vi "Main.vi"() -> ()   [LabVIEW 2013]
uses:
  Control 1.ctl
  Moteurs PI/PI Controls/Type de Mouvement PI.ctl
  Moteurs PI/PI Controls/AxeADeplacer.ctl
  PilMOT/Controls/Axes.ctl
  Commandes/Type de Mouvement PilMOT.ctl
  Moteurs PI/PI Globals/Zero.vi
panel:
  out "INIT":bool caption="En cours..."
  in  "CLR ERR mot PI 2":bool
  out "error out \nPI Enceinte 2":errorcluster
  in  "Fichier Fins de Courses":path=path "C:/Users/appli/Documents/Manip Gaz/Moteurs manip Gaz - Multithread/PilMOT/RefsMoteurs/FDC.dat"
  in  "CLR ERR mot PI":bool
  out "error out \nPI Enceinte":errorcluster
  in  "CLR ERR LàR":bool
  out "error out\nLabview functions":errorcluster
  in  "Fichier zéro ligne à retard":path=path "C:/Users/appli/Documents/Manip Gaz/Moteurs manip Gaz - Multithread/Moteurs PI/PI Globals/zero.dat"
  out "error out \nligne à retard":errorcluster
  in  "stop":bool
  out "error out\nesbim":cluster{"status":bool, "code":i32, "source":T1}
  in  "Commande onglets":T2(tab)
  in  "Axes\nà ref. 2":string[](array[string])=["1", "2", "3", "4"]
  in  "Modèles des platines":string[](array[string])=["M-111.1VG ", "M-111.1VG ", "M-111.1VG ", "M-111.1VG "]
  in  "Referencing":T3={"Check FRF?"=TRUE, "Referencing mode"=[enum."FPL", enum."FPL", enum."FPL", enum."FPL", enum."FRF (-> FNL)", enum."FRF (-> FNL)"]}
  out "Referencing...":bool caption="En cours..."
  in  "Limit switch selection":u16[](array[ring]) items=["Positive (MPL)", "Negative (MNL)"]
  out "Host address":string
  out "Referencing\nsuccessful?":bool[](array[boolean])
  in  "Ref tous\nles axes? 2":bool=TRUE
  out "Amplitude \n (+/-) (mm) 2":dbl[](array[numeric]) format="%.6f"
  out "Position 2":dbl[](array[numeric]) format="%.6f"
  out "Referencing...":bool
  out "Etat moteurs PI Buse/Capillaire 2":string
  out "Axes \nConn. 2":string[](array[string])
  in  "Configurer moteurs Enceinte (PI) 2":bool
  out "Identification C884":string
  out "En cours... 2":bool
  in  "Configurer Mercury (PI)":bool
  out "Etat moteurs PI Capillaire/Objectif":string
  in  "Configurer moteurs Enceinte (PI)":bool
  out "Identification carte de contrôle":string
  out "Axes \nConn.":string[](array[string])
  out "Amplitude \ndu mouvement\npermise (+/-) (mm)":dbl[](array[numeric]) format="%.6f"
  in  "Déplacement \nmi-course?":bool
  in  "Axes\nà ref.":string[](array[string])=["1", "2", "3", "4"]
  in  "Ref tous\nles axes?":bool
  out "Position":dbl[](array[numeric]) format="%.6f"
  out "+/- movement\nrange":dbl[](array[numeric]) format="%.6f"
  out "Position ligne à retard":dbl[](array[numeric]) format="%.6f"
  out "Conn. \nAxes":string[](array[string])
  out "Identification":string
  out "Etat ligne à retard":string
  in  "Stage selection":T4
  out "Axes \nConnectés\n(PI)  2":string[](array[string])
  in  "Positions de référence 2":dbl[][](array[numeric])=[[0.0, 0.0, 0.0, 0.0], [0.0, 0.0, 0.0, 0.0], [0.0, 0.0, 0.0, 0.0], [0.0, 0.0, 0.0, 0.0]] format="%_7g"
  out "Axes \nConnectés\n(PI)":string[](array[string])
  in  "SafeMax 2":dbl[](array[numeric]) format="%.6f"
  in  "SafeMin 2":dbl[](array[numeric]) format="%.6f"
  in  "SafeMax 1":dbl[](array[numeric]) format="%.6f"
  in  "SafeMin 1":dbl[](array[numeric]) format="%.6f"
  out "Axe en MVT 2":bool[](array[boolean])
  out "Position Moteurs (PI) 2":dbl[](array[numeric]) format="%.6f"
  in  "Déplacement (mm) 2":dbl[](array[numeric]) format="%.6f"
  in  "Axes à déplacer \n(PI) 2":bool[](array[boolean])
  out "Initialisation OK? 2":bool
  out "Axe en MVT":bool[](array[boolean])
  in  "Stop Mvt":bool
  in  "Axe (PI refs)":T5
  in  "Axe à déplacer (PI)":T5
  in  "MVT+":bool
  in  "MVT-":bool
  in  "Référence":T6(ring)
  in  "Positions de référence":dbl[][](array[numeric])=[[0.0, 0.0, 0.0, 0.0], [0.0, 0.0, 0.0, 0.0], [0.0, 0.0, 0.0, 0.0], [0.0, 0.0, 0.0, 0.0]] format="%_7g"
  in  "Load":bool
  in  "Save":bool
  in  "Go to Ref (PI)":bool
  in  "Set Ref (PI)":bool
  in  "Axes à déplacer \n(PI)":bool[](array[boolean])
  in  "Type de déplacement":T7
  out "Position Moteurs (PI)":dbl[](array[numeric]) format="%.6f"
  in  "Déplacement (mm)":dbl[](array[numeric]) format="%.6f"
  in  "Déplacer":bool
  in  "Déplacement":dbl[](array[numeric])=[0.001]
  out "Initialisation OK?":bool
  in  "Nom Fichier Refs PI":string="REFS"
  in  "Stop here":bool
  out "Current zero position":dbl
  in  "zero":dbl
  in  "zero à :":bool
  in  "zero ici":bool
  in  "JOG + delay":bool
  in  "Go delay":bool
  in  "JOG -delay":bool
  in  "Delay to reach":dbl
  in  "Step Size (ps)":dbl
  out "Ligne à retard prête?":bool
  in  "JOG + position":bool
  in  "Go pos":bool
  in  "JOG - position":bool
  in  "Query Pos.":bool
  in  "Position à atteindre":dbl
  in  "Step Size (mm)":dbl
  out "Position de la ligne à retard":dbl(slide) min=-51.0 max=51.0 scale=0.0..100.0
  in  "Query Velocity":bool
  in  "Set Vel.":dbl
  in  "Set Velocity":bool
  out "Current velocity":dbl
  out "Error Description (delay line)":string
  out "Initialisation OK?":bool
  in  "Axe à déplacer PilMot":T8=1 items=["Axe 1"=1, "Axe 2"=2, "Axe 3"=3, "Axe 4"=4, "Axe 5"=5, "Axe 6"=6]
  in  "Positions de référence PilMot":dbl[][](array[numeric])=[[0.0, 0.0, 0.0, 0.0], [0.0, 0.0, 0.0, 0.0], [0.0, 0.0, 0.0, 0.0], [0.0, 0.0, 0.0, 0.0]] format="%_7g"
  in  "Nom Fichier Refs PilMOT":string="StepperRef"
  out "Envoi cmde PilMot?":bool
  in  "STOP MOTEURS!!":bool
  in  "Coeff µm/pas":dbl[](array[numeric])=[3.1, 3.1, 3.1, 3.1, 3.1, 3.1]
  out "Positons Moteurs":dbl[](array[numeric])
  in  "Mouvement Rel/Abs":u16(ring) items=["Mouvement Absolu", "Mouvement Relatif"]
  in  "Origine":bool
  in  "Vitesses":i32[](array[numeric])=[0, 0, 0, 0, 0, 0]
  in  "Axes à déplacer \n(PilMot)":bool[](array[boolean])
  in  "Aller à CàA":bool
  in  "Axe à déplacer":u16(ring)=1 items=["Axe 1"=1, "Axe 2"=2, "Axe 3"=3, "Axe 4"=4, "Axe 5"=5, "Axe 6"=6]
  in  "Déplacement -":bool
  in  "Déplacement +":bool
  out "Adresse du PilMOT":string="ni.var.psp://localhost/OPC/OPC1/esbimETH_1"
  in  "Cotes à atteindre":dbl[](array[numeric])=[0.0, 0.0, 0.0, 0.0, 0.0, 0.0] format="%_6f"
  in  "Connected?":bool
  in  "Référence PilMot":T6(ring)
  in  "Set Ref (PilMot)":bool
  in  "Go to Ref (PilMot)":bool
  in  "Save Ref PilMot":bool
  in  "Load Ref PilMot":bool
  # "NE JAMAIS REFERENCER EN POSITION OBJECTIF"
  # "Objective Focus"
  # "Objective height"
  # "Target Height"
  # "<unassigned>"
  # "Target Transverse"
  # "Target  Focus"
  # "Mitu Obj Focus"
  # "Mitu Obj Transverse"
  # "FNL"
  # "FPL"
  # "FNL"
  # "FPL"
  # "Objective Focus"
  # "Objective height"
  # "Target Height"
  # "<unassigned>"
  # "Target Transverse"
  # "Target  Focus"
  # "Mitu Obj Focus"
  # "Mitu Obj Transverse"
  # "Objective Focus"
  # "Objective height"
  # "Target Height"
  # "<unassigned>"
  # "Target Transverse"
  # "Target  Focus"
  # "<unassigned>"
  # "<unassigned>"
  # "mm"
  # "mm"
  # "Spectro Electrons"
  # "NO MOTOR"
  # "Objectif/Jet"
  # "Pinhole Spectro"
  # "Parabole reprise"
  # "HeNe Salle Orange"
  # "Moteur 1"
  # "Spectro Electrons"
  # "Objectif/Jet"
  # "Pinhole Spectro"
  # "Parabole reprise"
  # "Moteur 6"
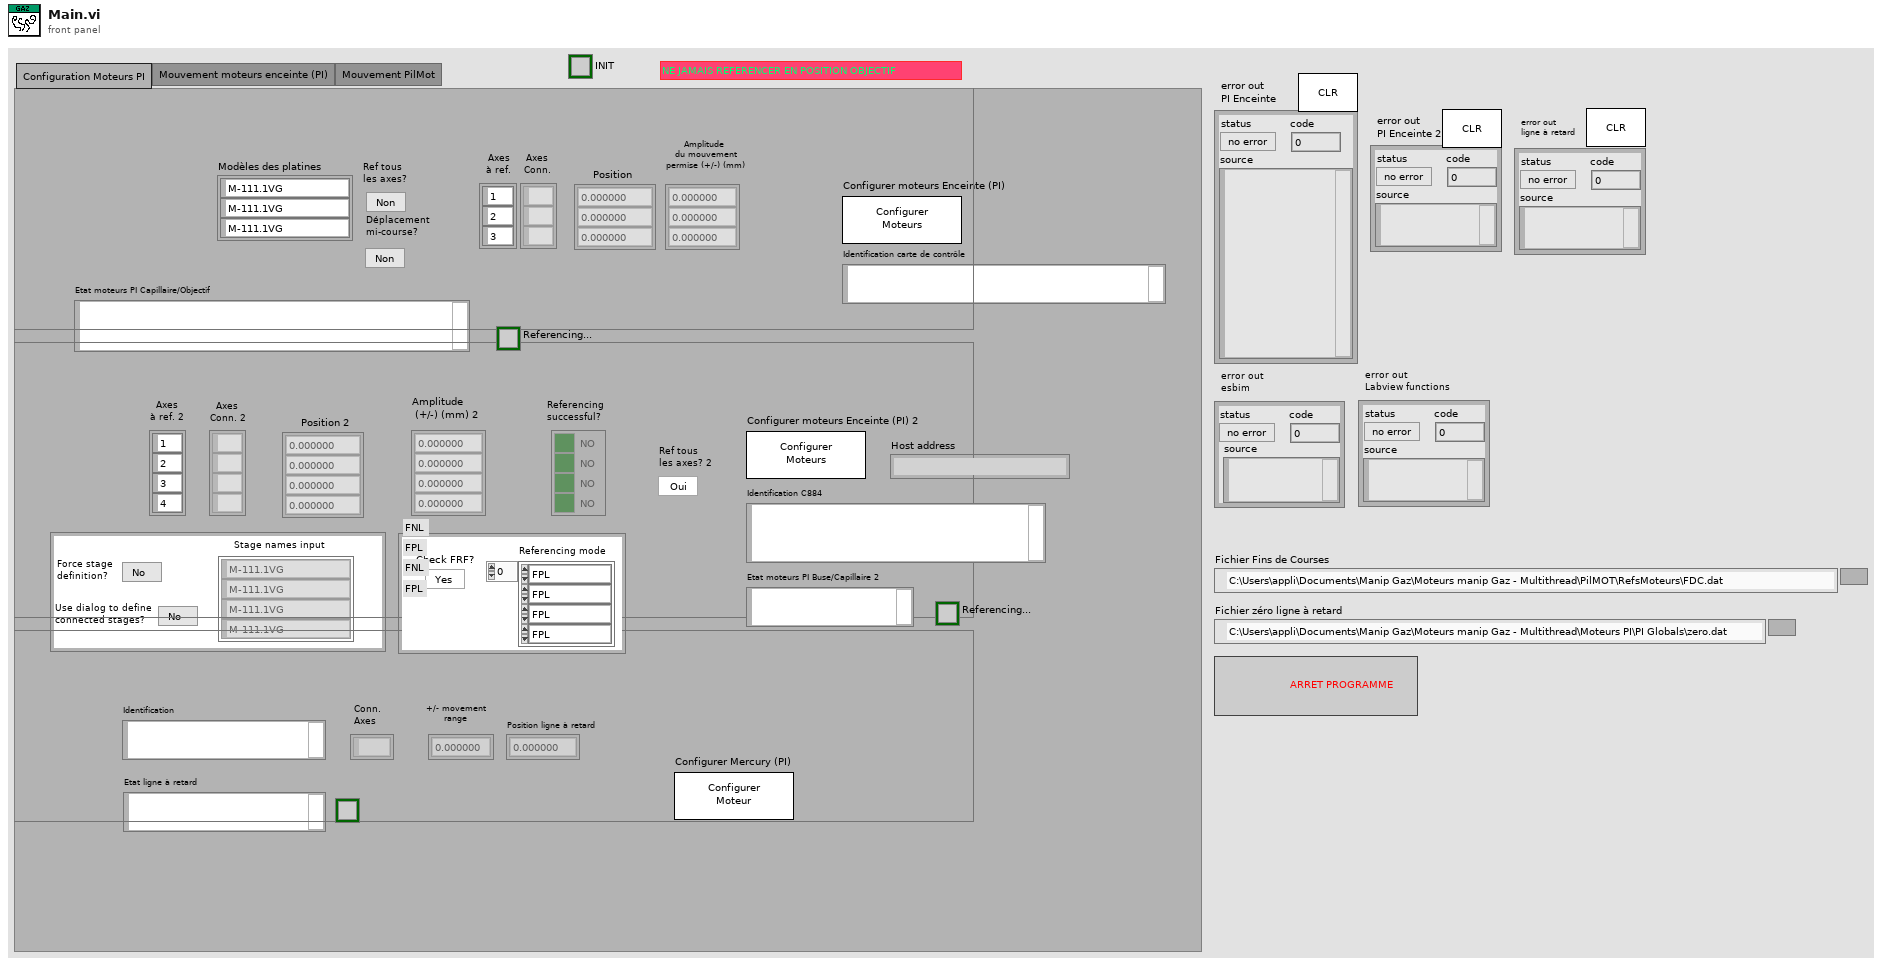
[diagram p1: front panel]
types:
  T1 = typedef "Control 1.ctl" = string
  T2 = enum32{"Configuration Moteurs PI", "Mouvement moteurs enceinte (PI)", "Mouvement Ligne à retard (PI)", "Mouvement PilMot"}
  T3 = cluster{"Check FRF?":bool, "Referencing mode":enum16{"FRF (-> FNL)", "FRF", "FNL", "FPL", "RON OFF"}[]}
  T4 = cluster{"Force?":bool, "Dialog?":bool, "Stages":string[]}
  T5 = typedef "AxeADeplacer.ctl" = enum16{"Objective Focus", "Objective Height", "Target Height", "<unassigned 1, 4>", "Target Transverse", "Target Focus", "Mitu Obj Focus", "Mitu Obj Transverse"}
  T6 = enum16{"Référence 1", "Référence 2", "Référence 3", "Référence 4"}
  T7 = typedef "Type de Mouvement PI.ctl" = enum16{"Mouvement absolu", "Mouvement relatif (-)", "Mouvement relatif (+)", "Définir pos. référence", "Aller à la pos. ref."}
  T8 = typedef "Axes.ctl" = u16
  T9 = enum16{"open", "replace", "create", "open or create", "replace or create", "replace or create with confirmation"}
  T10 = typedef "Type de Mouvement PilMOT.ctl" = u16
  T11 = typedef "AdressesVariablesPartagees.ctl" = cluster{"OrdreBloc":string, "Ordre UC":string, "CoteAAtteindre":string, "Vitesse":string, "Position codeur en pas":string, "Position Théorique":string, "Message":string, "Ecrire":string, "Zone à écrire":string, "Numéro paramètre":string, "Ordre":string, "Valeur":string, "Valeur Lecture":string, "Numéro paramètre Lecture":string, "Acquittement Lecture Ecriture":string, "Zone à Ecrire Pour Axe ":u16, "Acquittement Ordre UC":string}
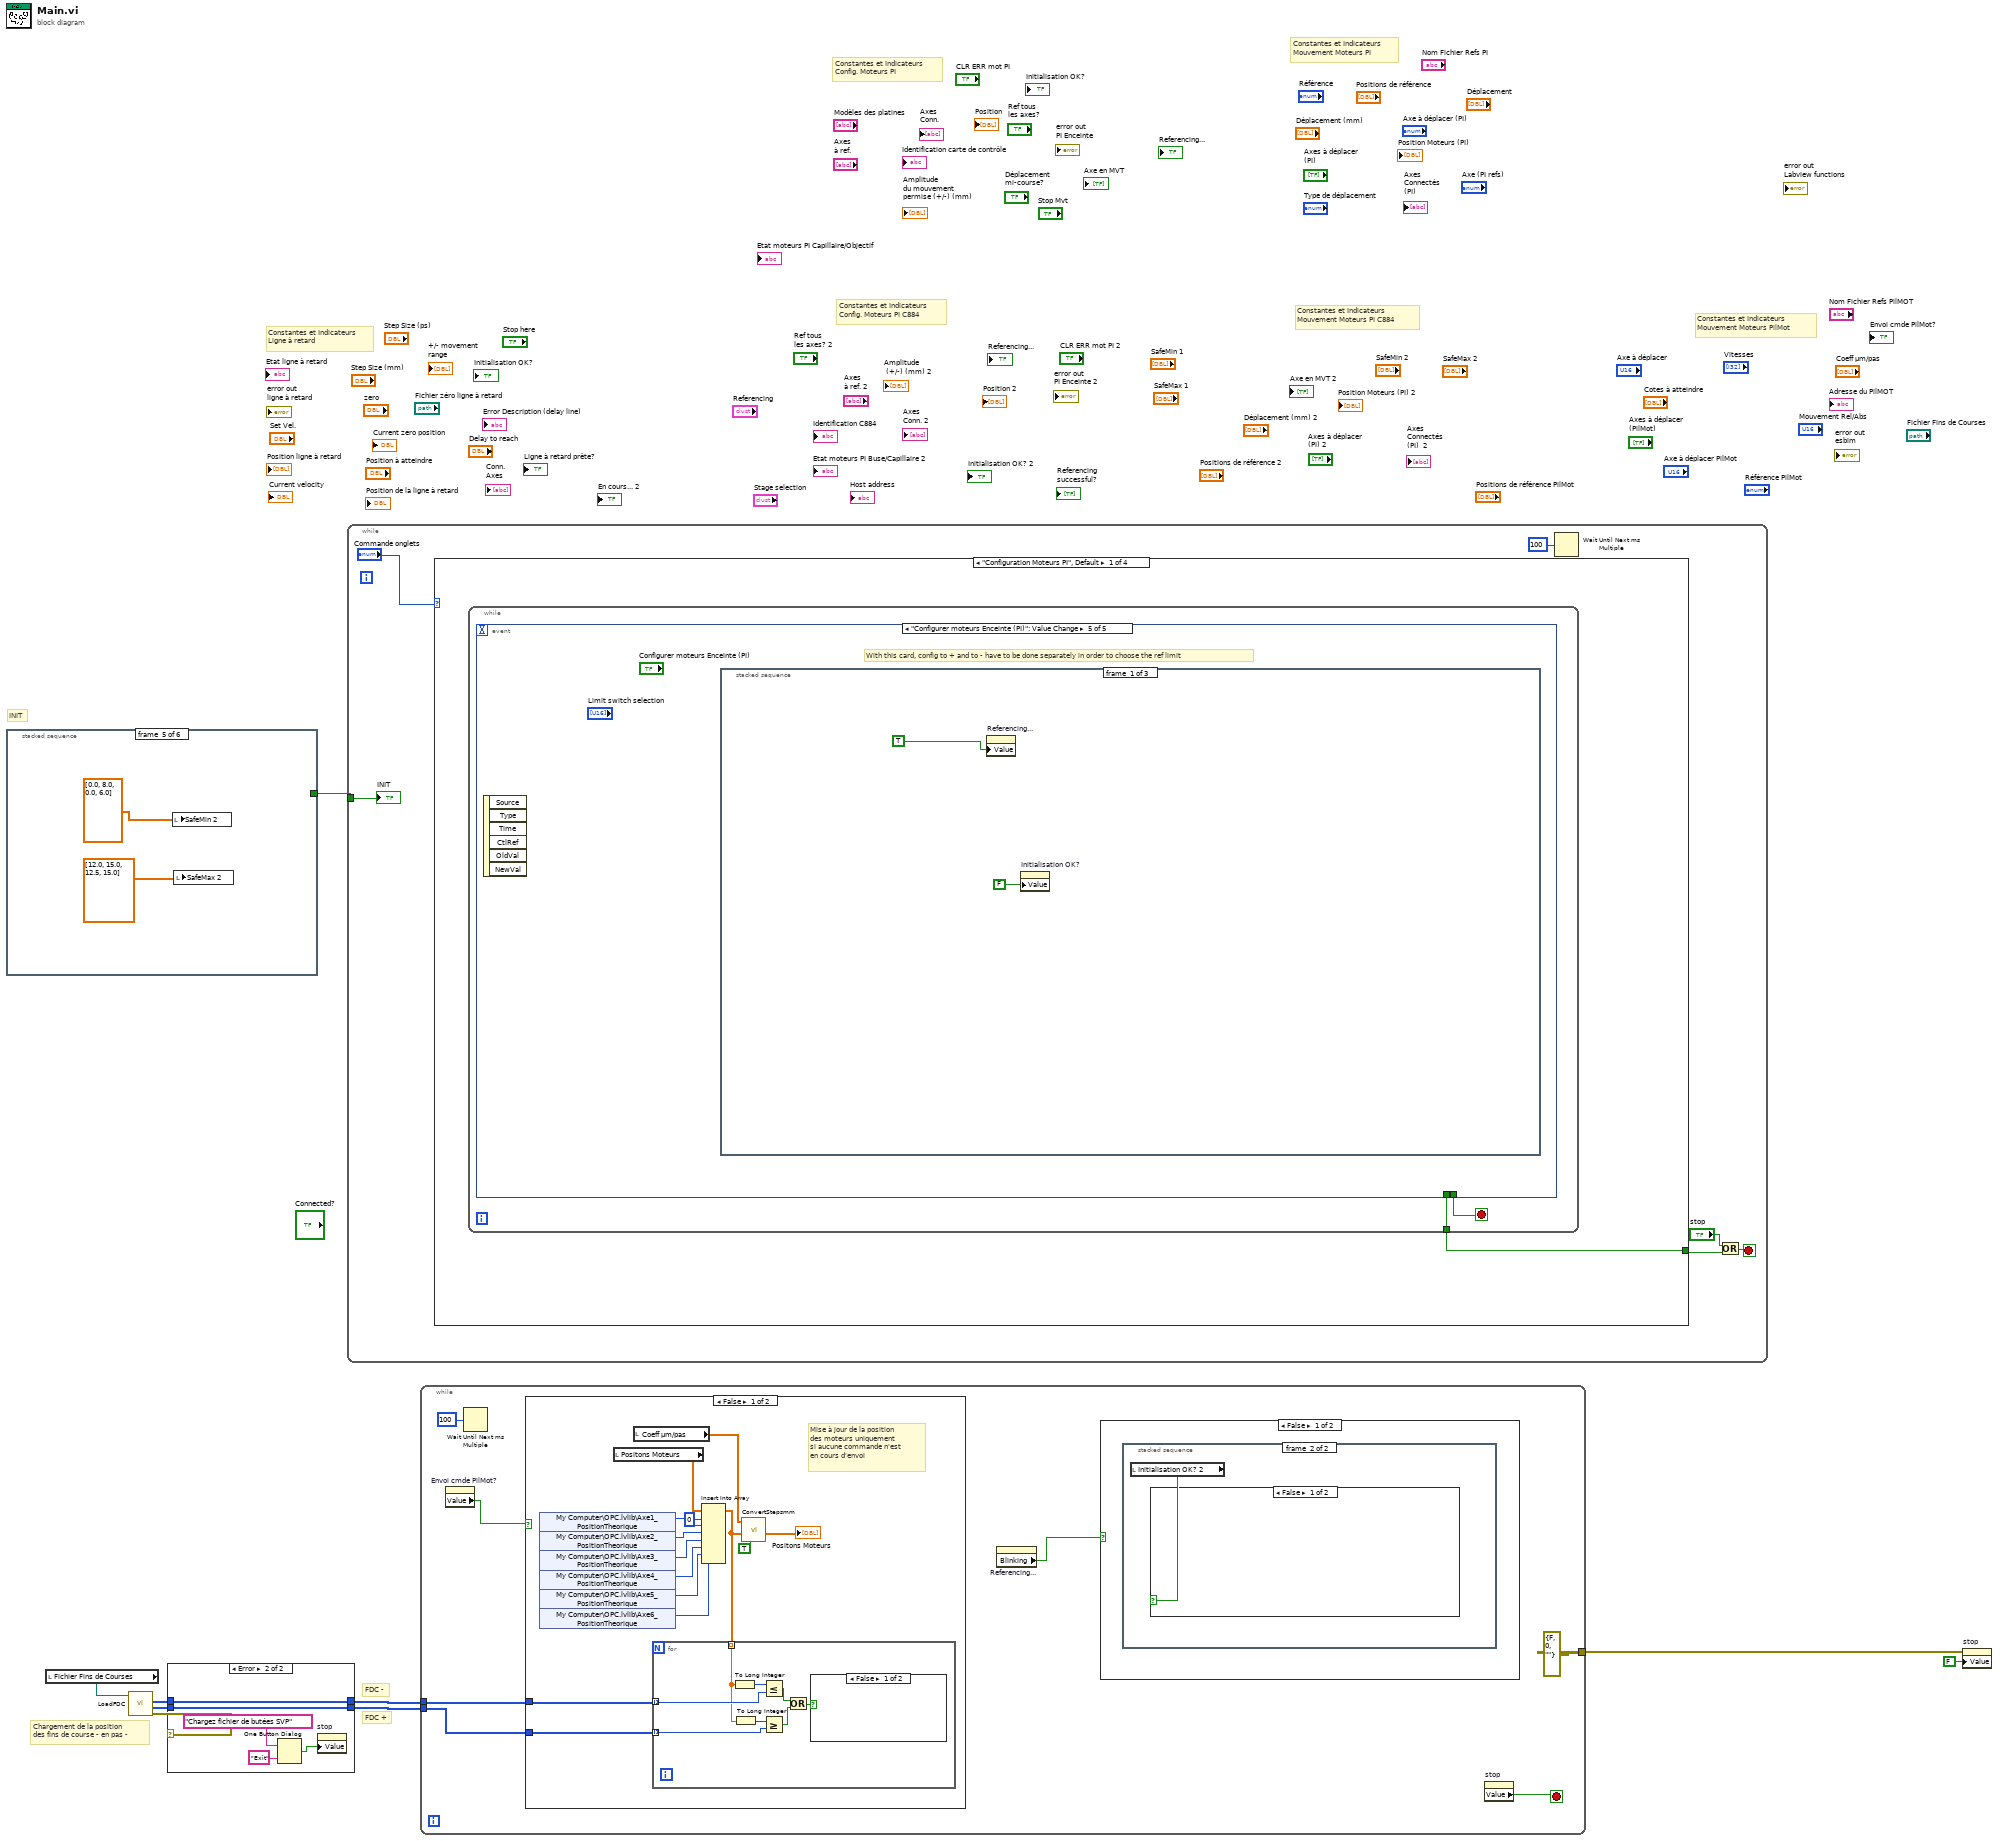
[diagram p0: block diagram]
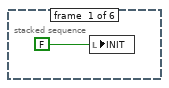
[diagram p2: hidden frame]
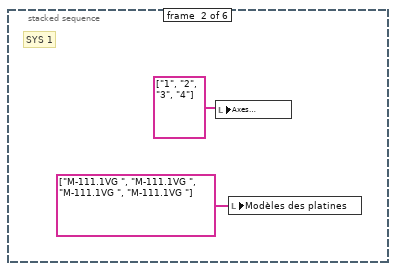
[diagram p3: hidden frame]
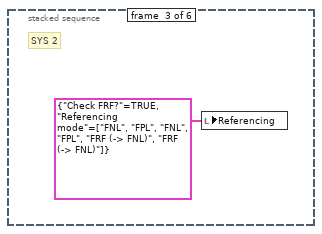
[diagram p4: hidden frame]
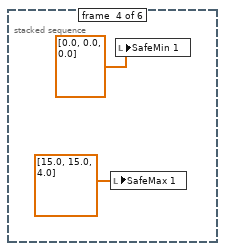
[diagram p5: hidden frame]
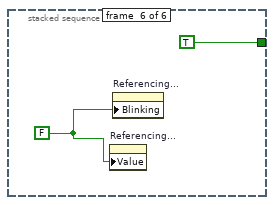
[diagram p6: hidden frame]
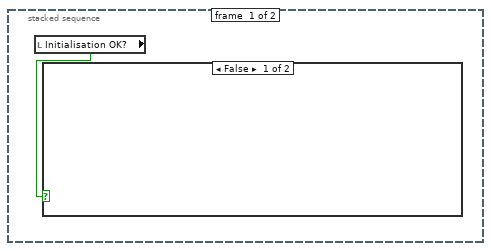
[diagram p8: hidden frame]
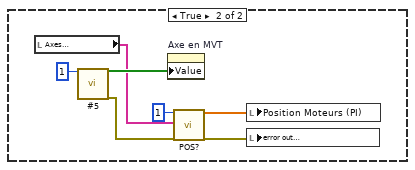
[diagram p9: hidden frame]
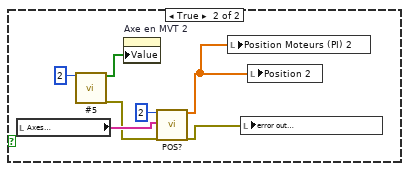
[diagram p10: hidden frame]
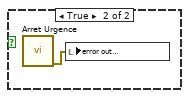
[diagram p12: hidden frame]
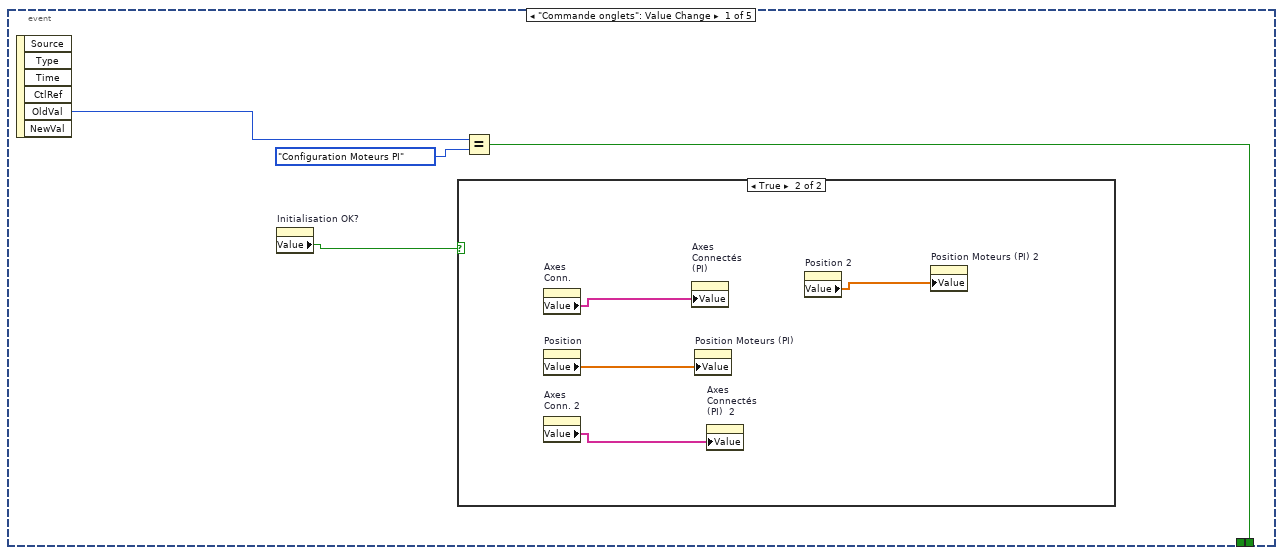
[diagram p14: hidden frame]
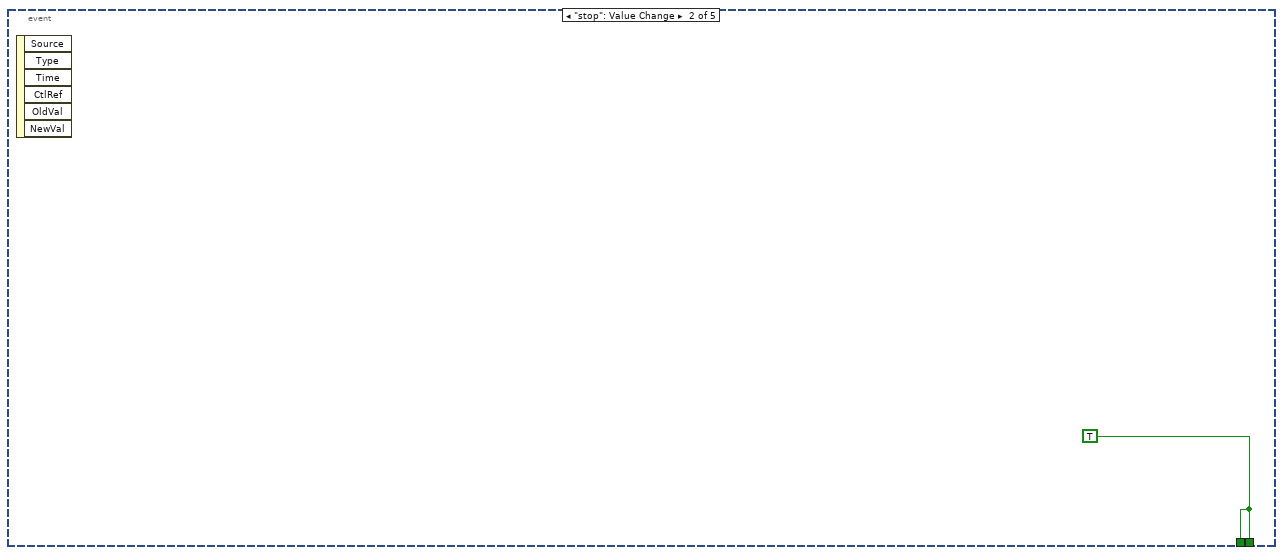
[diagram p16: hidden frame]
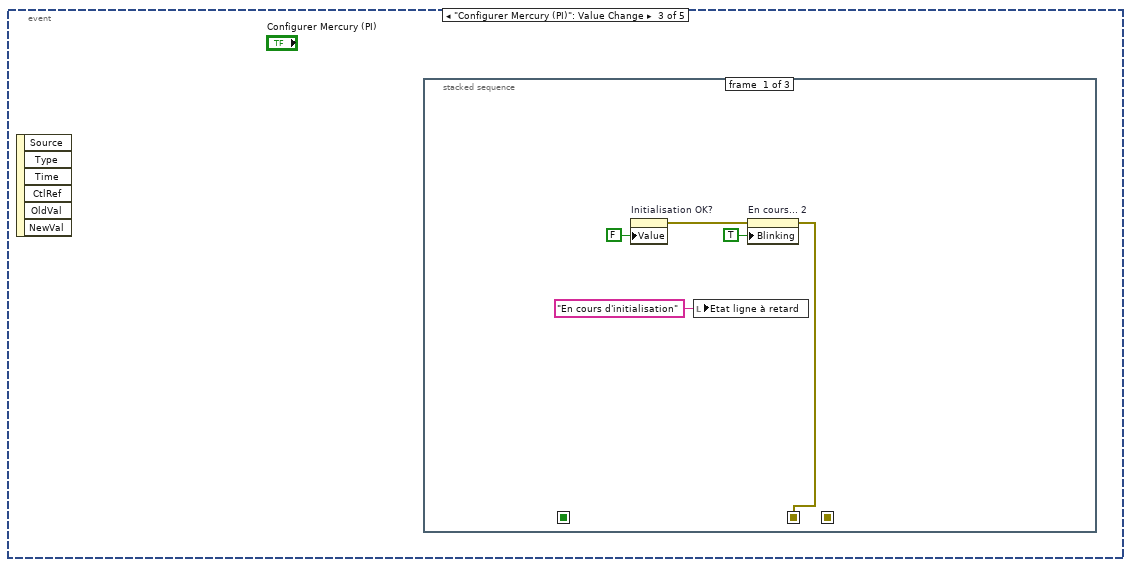
[diagram p17: hidden frame]
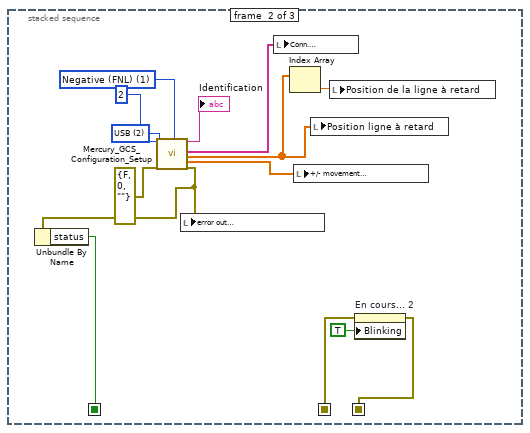
[diagram p18: hidden frame]
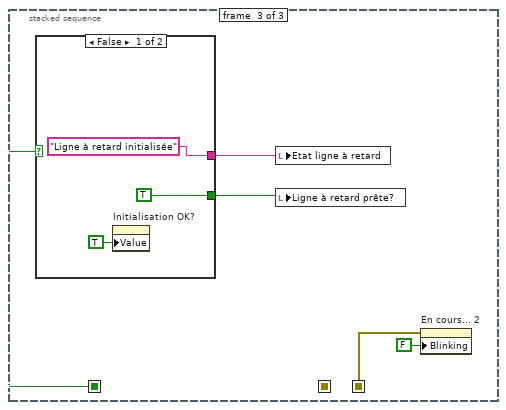
[diagram p19: hidden frame]
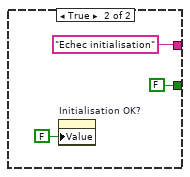
[diagram p20: hidden frame]
diagram:
  # "INIT"
  # "Constantes et Indicateurs\nMouvement Moteurs PI C884"
  # "Constantes et Indicateurs \nConfig. Moteurs PI C884"
  # "Chargement de la position \ndes fins de course - en pas -"
  # "FDC +"
  # "FDC -"
  # "Constantes et Indicateurs\nLigne à retard"
  # "Constantes et Indicateurs\nMouvement Moteurs PilMot"
  # "Constantes et Indicateurs\nMouvement Moteurs PI"
  # "Constantes et Indicateurs \nConfig. Moteurs PI"
  n1 = stacked-sequence {
    tunnel: [_ _ _ _ _ TRUE] -> w1
    frame #0 {
      n2 = local write "INIT"(FALSE) -> ()
    }
    frame #1 {
      # "SYS 1"
      n3 = local write "Axes\nà ref."(string[] ["1", "2", "3", "4"] ("Axes\nà ref.")) -> ()
      n4 = local write "Modèles des platines"(string[] ["M-111.1VG ", "M-111.1VG ", "M-111.1VG ", "M-111.1VG "] ("Modèles des platines")) -> ()
    }
    frame #2 {
      # "SYS 2"
      n5 = local write "Referencing"(T3 {"Check FRF?"=TRUE, "Referencing mode"=[enum."FNL", enum."FPL", enum."FNL", enum."FPL", enum."FRF (-> FNL)", enum."FRF (-> FNL)"]} ("Referencing")) -> ()
    }
    frame #3 {
      n6 = local write "SafeMax 1"(dbl[] [15.0, 15.0, 4.0] ("SafeMin 1")) -> ()
      n7 = local write "SafeMin 1"(dbl[] [0.0, 0.0, 0.0] ("SafeMin 1")) -> ()
    }
    frame #4 {
      n8 = local write "SafeMin 2"(dbl[] [0.0, 8.0, 0.0, 6.0] ("SafeMin 1")) -> ()
      n9 = local write "SafeMax 2"(dbl[] [12.0, 15.0, 12.5, 15.0] ("SafeMin 1")) -> ()
    }
    frame #5 {
      w18 = FALSE ("Blinking")
      n10 = property on="Referencing..." class="Bool (strict)"("Value"=w18) -> ()  [unwired: 2 in, 2 out]
      n11 = property on="Referencing..." class="Bool (strict)"("Blinking"=w18) -> ()  [unwired: 2 in, 2 out]
    }
  }
  n12 = local read "Fichier Fins de Courses"() -> (w7:path)
  n13 = call "LoadFDC.vi"("file path (use dialog)"=w7) -> ("error out"=w6:errorcluster, "FDC+"=w4:i32[], "FDC-"=w5:i32[])  [unwired: 8 in]
  n14 = case shown="Error" w6 {
    tunnel: w5 -> [w21 w26]
    tunnel: [w21 w26] -> w3
    tunnel: w4 -> [w20 w25]
    tunnel: [w20 w25] -> w2
    frame No Error {
    }
    frame Error {
      n15 = One Button Dialog(message="Chargez fichier de butées SVP", button name ("OK")="Exit") -> (true=w22:bool)
      n16 = property on="stop" class="Bool (strict)"("Value"=w22) -> ()  [unwired: 2 in, 2 out]
    }
  }
  n17 = while {
    tunnel: w1 -> [w27]
    stop <- w31 stop-if-true
    n18 = case shown="\"Configuration Moteurs PI\", Default" "Commande onglets" {
      tunnel: [w33 w123 w410 w577] -> w29
      frame "Configuration Moteurs PI", Default {
        n19 = while {
          tunnel: [w34] -> w33
          stop <- w35 stop-if-true
          n20 = event shown="[4] \"Configurer moteurs Enceinte (PI)\": Value Change" {
            selector: _ -> [_ _ _ _ _]
            dyn-events: _ -> [_ _ _ _ _]
            timeout: _ -> [_ _ _ _ _]
            tunnel: [w37 w44 _ _ _] -> w35
            tunnel: [_ w44 _ _ _] -> w34
            event "Commande onglets": Value Change {
              n21 = event-data() -> ("OldVal"=w39:T2)  [unwired: 1 in, 5 out]
              n22 = property on="Initialisation OK?" class="Bool (strict)"() -> ("Value"=w36:bool)  [unwired: 2 in, 2 out]
              n23 = case shown="True" w36 {
                frame False {
                }
                frame True {
                  n24 = property on="Axes \nConn." class="Arr (strict)"() -> ("Value"=w43:string[])  [unwired: 2 in, 2 out]
                  n25 = property on="Position" class="Arr (strict)"() -> ("Value"=w42:dbl[])  [unwired: 2 in, 2 out]
                  n26 = property on="Axes \nConn. 2" class="Arr (strict)"() -> ("Value"=w41:string[])  [unwired: 2 in, 2 out]
                  n27 = property on="Axes \nConnectés\n(PI)" class="Arr (strict)"("Value"=w43) -> ()  [unwired: 2 in, 2 out]
                  n28 = property on="Position Moteurs (PI)" class="Arr (strict)"("Value"=w42) -> ()  [unwired: 2 in, 2 out]
                  n29 = property on="Axes \nConnectés\n(PI)  2" class="Arr (strict)"("Value"=w41) -> ()  [unwired: 2 in, 2 out]
                  n30 = property on="Position 2" class="Arr (strict)"() -> ("Value"=w40:dbl[])  [unwired: 2 in, 2 out]
                  n31 = property on="Position Moteurs (PI) 2" class="Arr (strict)"("Value"=w40) -> ()  [unwired: 2 in, 2 out]
                }
              }
              n32 = Equal?(x=w39, y=T2."Configuration Moteurs PI" ("Commande onglets")) -> (x = y?=w37:bool)
            }
            event "stop": Value Change {
              w44 = TRUE
              n33 = event-data() -> ()  [unwired: 1 in, 6 out]
            }
            event "Configurer Mercury (PI)": Value Change {
              n34 = event-data() -> ()  [unwired: 1 in, 6 out]
              n35 = stacked-sequence {
                seq-local: [_ w57 _] -> [_ _ w68]
                seq-local: [w45 _ _] -> [_ w51 _]
                seq-local: [_ w50 _] -> [_ _ w64]
                frame #0 {
                  n36 = property on="Initialisation OK?" class="Bool (strict)"("Value"=FALSE ("Initialisation 2")) -> (error out=w46:errorcluster)  [unwired: 2 in, 1 out]
                  n37 = local write "Etat ligne à retard"("En cours d'initialisation" ("Etat ligne à retard")) -> ()
                  n38 = property on="En cours... 2" class="Bool (strict)"(error in=w46, "Blinking"=TRUE) -> (error out=w45:errorcluster)  [unwired: 1 in, 1 out]
                }
                frame #1 {
                  w60 = u16 1 items=["Positive (FPL)", "Negative (FNL)"] ("Limit switch selection")
                  w61 = u16 2 items=["RS232", "RS232 DaisyChain", "USB", "USB_DaisyChain"] ("Interface")
                  n39 = call "Mercury_GCS_Configuration_Setup.vi"("System no."=2, "Interface"=w61, "error in"=errorcluster {"status"=FALSE, "code"=0, "source"=""}, "Reference Move"=w60) -> ("Identification"=→"Identification":string, "Conn. \nAxes"=w56:string[], "Position"=w53:dbl[], "+/- movement\nrange"=w55:dbl[], "error out"=w58:errorcluster)  [unwired: 9 in, 2 out]
                  n40 = Unbundle By Name(w58) -> ("status"=w57:bool)
                  n41 = local write "error out \nligne à retard"(w58) -> ()
                  n42 = local write "Conn. \nAxes"(w56) -> ()
                  n43 = Index Array(array=w53) -> (element=w54:dbl)  [unwired: 1 in]
                  n44 = local write "+/- movement\nrange"(w55) -> ()
                  n45 = local write "Position ligne à retard"(w53) -> ()
                  n46 = local write "Position de la ligne à retard"(w54) -> ()
                  n47 = property on="En cours... 2" class="Bool (strict)"(error in=w51, "Blinking"=TRUE) -> (error out=w50:errorcluster)  [unwired: 1 in, 1 out]
                }
                frame #2 {
                  n48 = case shown="False" w68 {
                    tunnel: ["Ligne à retard initialisée" ("Etat ligne à retard") "Echec initialisation" ("Etat ligne à retard")] -> w67
                    tunnel: [TRUE FALSE] -> w66
                    frame False {
                      n49 = property on="Initialisation OK?" class="Bool (strict)"("Value"=TRUE ("Initialisation 2")) -> ()  [unwired: 2 in, 2 out]
                    }
                    frame True {
                      n50 = property on="Initialisation OK?" class="Bool (strict)"("Value"=FALSE ("Initialisation 2")) -> ()  [unwired: 2 in, 2 out]
                    }
                  }
                  n51 = local write "Etat ligne à retard"(w67) -> ()
                  n52 = local write "Ligne à retard prête?"(w66) -> ()
                  n53 = property on="En cours... 2" class="Bool (strict)"(error in=w64, "Blinking"=FALSE) -> ()  [unwired: 1 in, 2 out]
                }
              }
            }
            event "Configurer moteurs Enceinte (PI) 2": Value Change {
              n54 = event-data() -> ()  [unwired: 1 in, 6 out]
              n55 = stacked-sequence {
                frame #0 {
                  n56 = property on="Initialisation OK? 2" class="Bool (strict)"("Value"=FALSE ("Initialisation OK? 2")) -> ()  [unwired: 2 in, 2 out]
                  n57 = property on="Referencing..." class="Bool (strict)"("Value"=TRUE ("Blinking")) -> ()  [unwired: 2 in, 2 out]
                  n58 = local write "Etat moteurs PI Buse/Capillaire 2"("Initialisation en cours, \npatientez...") -> ()
                }
                frame #1 {
                  n59 = local read "Stage selection"() -> (w79:T4)
                  n60 = control-ref of="Identification C884"() -> (w92:refnum<vi>)
                  n61 = control-ref of="Position 2"() -> (w93:refnum<vi>)
                  n62 = control-ref of="Referencing\nsuccessful?"() -> (w91:refnum<vi>)
                  n63 = control-ref of="Host address"() -> (w90:refnum<vi>)
                  n64 = vi-ref "C884Config.vi"() -> (w98:refnum<vi>)
                  n65 = local read "Referencing"() -> (w78:T3)
                  n66 = control-ref of="Ref tous\nles axes? 2"() -> (w94:refnum<vi>)
                  n67 = control-ref of="Etat moteurs PI Buse/Capillaire 2"() -> (w81:refnum<vi>)
                  n68 = control-ref of="Initialisation OK? 2"() -> (w82:refnum<vi>)
                  n69 = property class="VI"(reference=w98) -> ("Name"=w97:string)  [unwired: 1 in, 2 out]
                  n70 = control-ref of="Amplitude \n (+/-) (mm) 2"() -> (w89:refnum<vi>)
                  n71 = control-ref of="Axes \nConn. 2"() -> (w88:refnum<vi>)
                  n72 = Open VI Reference(type specifier VI Refnum (for type only)=refnum<vi> refnum, vi path=w97, options=128) -> (vi reference=w95:refnum<vi>, error out=w84:errorcluster)  [unwired: 3 in]
                  n73 = control-ref of="error out \nPI Enceinte 2"() -> (w87:refnum<vi>)
                  n74 = control-ref of="Axes\nà ref. 2"() -> (w86:refnum<vi>)
                  n75 = control-ref of="Referencing..."() -> (w80:refnum<vi>)
                  n76 = call-by-ref "Start Asynchronous Call"(reference=w95, error in=w84, "All axes? Refnum"=w94, "Stage selection"=w79, "Position Refnum"=w93, "Identification Refnum"=w92, "Referencing successful Refnum"=w91, "Host Addresss Refnum"=w90, "Message Out Refnum"=w81, "+/- mvt range Refnum"=w89, "Axes to Move Refnum"=w86, "Connected Axes Refnum"=w88, "Referencing"=w78, "Error OUT Refnum"=w87, "En cours LED Refnum"=w80, "LED Initialis. OK? Refnum"=w82) -> (reference out=w85:refnum<vi>, error out=w83:errorcluster)  [unwired: 6 in]
                  n77 = Close Reference(reference=w85, error in (no error)=w83) -> ()  [unwired: 1 out]
                }
                frame #2 {
                  n78 = property on="Referencing..." class="Bool (strict)"("Value"=FALSE ("Blinking")) -> ()  [unwired: 2 in, 2 out]
                }
              }
            }
            event "Configurer moteurs Enceinte (PI)": Value Change {
              # "With this card, config to + and to - have to be done separately in order to choose the ref limit"
              n79 = event-data() -> ()  [unwired: 1 in, 6 out]
              n80 = stacked-sequence {
                frame #0 {
                  n81 = property on="Referencing..." class="Bool (strict)"("Value"=TRUE ("Initialisation OK?")) -> ()  [unwired: 2 in, 2 out]
                  n82 = property on="Initialisation OK?" class="Bool (strict)"("Value"=FALSE ("Initialisation OK?")) -> ()  [unwired: 2 in, 2 out]
                }
                frame #1 {
                  # "Subarray with positive referencing"
                  # "Positive reference"
                  n83 = vi-ref "C843Config.vi"() -> (w106:refnum<vi>)
                  n84 = property class="VI"(reference=w106) -> ("Name"=w119:string)  [unwired: 1 in, 2 out]
                  n85 = Open VI Reference(type specifier VI Refnum (for type only)=refnum<vi> refnum, vi path=w119, options=128) -> (vi reference=w120:refnum<vi>)  [unwired: 3 in, 1 out]
                  n86 = local read "Axes\nà ref."() -> (w104:string[])
                  n87 = control-ref of="Amplitude \ndu mouvement\npermise (+/-) (mm)"() -> (w118:refnum<vi>)
                  n88 = control-ref of="Modèles des platines"() -> (w114:refnum<vi>)
                  n89 = control-ref of="error out \nPI Enceinte"() -> (w111:refnum<vi>)
                  n90 = control-ref of="Identification carte de contrôle"() -> (w113:refnum<vi>)
                  n91 = control-ref of="Etat moteurs PI Capillaire/Objectif"() -> (w110:refnum<vi>)
                  n92 = control-ref of="Axes \nConn."() -> (w117:refnum<vi>)
                  n93 = control-ref of="Initialisation OK?"() -> (w116:refnum<vi>)
                  n94 = control-ref of="Position"() -> (w112:refnum<vi>)
                  n95 = control-ref of="Ref tous\nles axes?"() -> (w115:refnum<vi>)
                  n96 = control-ref of="Referencing..."() -> (w103:refnum<vi>)
                  n97 = call-by-ref "Start Asynchronous Call"(reference=w120, "Axes to Move"=w104, "Initialisation OK Refnum"=w116, "All Axes? Refnum"=w115, "Stage names Input Refnum"=w114, "Identification Refnum"=w113, "Connected Axes Refnum"=w117, "Position Refnum"=w112, "+/- movement range Refnum"=w118, "Error Out Refnum"=w111, "LED status Refnum"=w103, "Etat moteurs Refnum"=w110) -> (reference out=w108:refnum<vi>, error out=w109:errorcluster)  [unwired: 10 in]
                  n98 = Close Reference(reference=w108, error in (no error)=w109) -> (error out=w107:errorcluster)
                  n99 = call <vilib>:"Simple Error Handler.vi"("error in (no error)"=w107) -> ()  [unwired: 4 in, 5 out]
                }
                frame #2 {
                  n100 = property on="Referencing..." class="Bool (strict)"("Value"=FALSE ("Initialisation OK?")) -> ()  [unwired: 2 in, 2 out]
                }
              }
            }
          }
        }
      }
      frame "Mouvement moteurs enceinte (PI)" {
        n101 = while {
          tunnel: [w125] -> w123
          stop <- w124 stop-if-true
          n102 = event shown="[5] \"Save\": Value Change" {
            selector: _ -> [_ _ _ _ _ _ _ _ _]
            dyn-events: _ -> [_ _ _ _ _ _ _ _ _]
            timeout: _ -> [_ _ _ _ _ _ _ _ _]
            tunnel: [_ _ _ _ _ _ w395 _ _] -> w125
            tunnel: [_ _ _ _ _ _ w395 w396 _] -> w124
            event "Déplacer": Value Change {
              n103 = event-data() -> ()  [unwired: 1 in, 6 out]
              n104 = stacked-sequence {
                frame #0 {
                  # "Set de moteurs #1"
                  n105 = stacked-sequence {
                    seq-local: [_ w136 _ _] -> [_ _ w141 _]
                    seq-local: [_ w135 _ _] -> [_ _ w142 _]
                    seq-local: [w127 _ _ _] -> [_ w134 _ _]
                    seq-local: [_ w133 _ _] -> [_ _ w139 _]
                    tunnel: [_ _ w140 _] -> w126
                    frame #0 {
                      n106 = local read "Axes \nConnectés\n(PI)"() -> (w131:string[])
                      n107 = local read "Axes à déplacer \n(PI)"() -> (w129:bool[])
                      n108 = local read "Déplacement (mm)"() -> (w130:dbl[])
                      n109 = call "ReduceToConnectedAxes.vi"("Axes à déplacer input"=w129, "Déplacements input"=w130, "Axes connectés"=w131) -> ("Axes à déplacer output"=w128:bool[], "Déplacements output"=w127:dbl[])  [unwired: 7 in]
                      n110 = local write "Axes à déplacer \n(PI)"(w128) -> ()
                    }
                    frame #1 {
                      n111 = local read "Axes à déplacer \n(PI)"() -> (w138:bool[])
                      n112 = local read "Axes \nConnectés\n(PI)"() -> (w137:string[])
                      n113 = call "ArraySearchWhichMove.vi"("System n°"=u16 1, "Tableau d'axes connectés"=w137, "Tableau de déplacements input"=w134, "Tableau d'axes à déplacer input"=w138) -> ("Mvt des moteurs"=w133:bool, "Tableau d'axes à déplacer output"=w136:string[], "Tableau de déplacements output"=w135:dbl[])  [unwired: 4 in]
                    }
                    frame #2 {
                      n114 = case shown="True" w139 {
                        tunnel: w142 -> [_ w146]
                        tunnel: w141 -> [_ w145]
                        tunnel: [_ w144] -> w140
                        frame False {
                        }
                        frame True {
                          n115 = local read "Type de déplacement"() -> (w149:T7)
                          n116 = case shown="\"Mouvement absolu\", Default" w149 {
                            tunnel: [w158 w164 w168 w173 w178] -> w144
                            tunnel: 1 ("System no.") -> [w157 w165 w170 w174 w180]
                            tunnel: TRUE ("Move absolute") -> [w156 w162 w166 w175 w177]
                            tunnel: [w155 w163 w169 w172 w179] -> w143
                            tunnel: w145 -> [w154 w161 w167 w171 w176]
                            tunnel: w146 -> [w153 _ _ _ _]
                            frame "Mouvement absolu", Default {
                              n117 = local read "SafeMax 1"() -> (w151:dbl[])
                              n118 = local read "SafeMin 1"() -> (w150:dbl[])
                              n119 = control-ref of="Stop Mvt"() -> (w152:refnum<vi>)
                              n120 = call "MoveSinglePIMotor.vi"("System no."=w157, "Axes to move"=w154, "Move"=w153, "SafeMax"=w151, "SafeMin"=w150, "Move absolute"=w156, "Stop refnum"=w152) -> ("Position"=w155:dbl[], "error out"=w158:errorcluster)  [unwired: 11 in]
                            }
                            frame "Mouvement relatif (-)" {
                              n121 = local read "error out \nPI Enceinte"() -> (w160:errorcluster)
                              n122 = control-ref of="Stop Mvt"() -> (w159:refnum<vi>)
                              n123 = call "MoveSinglePIMotor.vi"("System no."=w165, "Axes to move"=w161, "error in"=w160, "Move relative (-)"=w162, "Stop refnum"=w159) -> ("Position"=w163:dbl[], "error out"=w164:errorcluster)  [unwired: 13 in]
                            }
                            frame "Mouvement relatif (+)" {
                              n124 = call "MoveSinglePIMotor.vi"("System no."=w170, "Axes to move"=w167, "Move relative (+)"=w166) -> ("Position"=w169:dbl[], "error out"=w168:errorcluster)  [unwired: 15 in]
                            }
                            frame "Définir pos. référence" {
                              n125 = call "MoveSinglePIMotor.vi"("System no."=w174, "Axes to move"=w171, "Go home"=w175) -> ("Position"=w172:dbl[], "error out"=w173:errorcluster)  [unwired: 15 in]
                            }
                            frame "Aller à la pos. ref." {
                              n126 = call "MoveSinglePIMotor.vi"("System no."=w180, "Axes to move"=w176, "Go home"=w177) -> ("Position"=w179:dbl[], "error out"=w178:errorcluster)  [unwired: 15 in]
                            }
                          }
                          n127 = shared-variable "My Computer\\PSP Variables Lib.lvlib\\Position Moteurs PI PSP"(w143) -> ()  [unwired: 1 in, 1 out]
                          n128 = local write "Position Moteurs (PI)"(w143) -> ()
                        }
                      }
                    }
                    frame #3 {
                      n129 = property on="Stop Mvt" class="Bool (strict)"("Value"=FALSE ("Stop Mvt")) -> ()  [unwired: 2 in, 2 out]
                    }
                  }
                  n130 = local write "error out \nPI Enceinte"(w126) -> ()
                }
                frame #1 {
                  # "Set de moteurs #2"
                  n131 = stacked-sequence {
                    seq-local: [_ w191 _ _] -> [_ _ w196 _]
                    seq-local: [_ w190 _ _] -> [_ _ w197 _]
                    seq-local: [w182 _ _ _] -> [_ w189 _ _]
                    seq-local: [_ w188 _ _] -> [_ _ w194 _]
                    tunnel: [_ _ w195 _] -> _
                    frame #0 {
                      n132 = local read "Axes \nConnectés\n(PI)  2"() -> (w186:string[])
                      n133 = local read "Axes à déplacer \n(PI) 2"() -> (w184:bool[])
                      n134 = local read "Déplacement (mm) 2"() -> (w185:dbl[])
                      n135 = call "ReduceToConnectedAxes.vi"("Axes à déplacer input"=w184, "Déplacements input"=w185, "Axes connectés"=w186) -> ("Axes à déplacer output"=w183:bool[], "Déplacements output"=w182:dbl[])  [unwired: 7 in]
                      n136 = local write "Axes à déplacer \n(PI) 2"(w183) -> ()
                    }
                    frame #1 {
                      n137 = local read "Axes \nConnectés\n(PI)  2"() -> (w192:string[])
                      n138 = local read "Axes à déplacer \n(PI) 2"() -> (w193:bool[])
                      n139 = call "ArraySearchWhichMove.vi"("System n°"=u16 2, "Tableau d'axes connectés"=w192, "Tableau de déplacements input"=w189, "Tableau d'axes à déplacer input"=w193) -> ("Mvt des moteurs"=w188:bool, "Tableau d'axes à déplacer output"=w191:string[], "Tableau de déplacements output"=w190:dbl[])  [unwired: 4 in]
                    }
                    frame #2 {
                      n140 = case shown="True" w194 {
                        tunnel: w197 -> [_ w201]
                        tunnel: w196 -> [_ w200]
                        tunnel: [_ w199] -> w195
                        frame False {
                        }
                        frame True {
                          n141 = local read "Type de déplacement"() -> (w204:T7)
                          n142 = case shown="\"Mouvement absolu\", Default" w204 {
                            tunnel: [w213 w219 w223 w228 w233] -> w199
                            tunnel: 2 ("System no.") -> [w212 w220 w225 w229 w235]
                            tunnel: TRUE ("Move absolute") -> [w211 w217 w221 w230 w232]
                            tunnel: [w210 w218 w224 w227 w234] -> w198
                            tunnel: w200 -> [w209 w216 w222 w226 w231]
                            tunnel: w201 -> [w208 _ _ _ _]
                            frame "Mouvement absolu", Default {
                              n143 = local read "SafeMax 2"() -> (w206:dbl[])
                              n144 = local read "SafeMin 2"() -> (w205:dbl[])
                              n145 = control-ref of="Stop Mvt"() -> (w207:refnum<vi>)
                              n146 = call "MoveSinglePIMotor.vi"("System no."=w212, "Axes to move"=w209, "Move"=w208, "SafeMax"=w206, "SafeMin"=w205, "Move absolute"=w211, "Stop refnum"=w207) -> ("Position"=w210:dbl[], "error out"=w213:errorcluster)  [unwired: 11 in]
                            }
                            frame "Mouvement relatif (-)" {
                              n147 = local read "error out \nPI Enceinte 2"() -> (w215:errorcluster)
                              n148 = control-ref of="Stop Mvt"() -> (w214:refnum<vi>)
                              n149 = call "MoveSinglePIMotor.vi"("System no."=w220, "Axes to move"=w216, "error in"=w215, "Move relative (-)"=w217, "Stop refnum"=w214) -> ("Position"=w218:dbl[], "error out"=w219:errorcluster)  [unwired: 13 in]
                            }
                            frame "Mouvement relatif (+)" {
                              n150 = call "MoveSinglePIMotor.vi"("System no."=w225, "Axes to move"=w222, "Move relative (+)"=w221) -> ("Position"=w224:dbl[], "error out"=w223:errorcluster)  [unwired: 15 in]
                            }
                            frame "Définir pos. référence" {
                              n151 = call "MoveSinglePIMotor.vi"("System no."=w229, "Axes to move"=w226, "Go home"=w230) -> ("Position"=w227:dbl[], "error out"=w228:errorcluster)  [unwired: 15 in]
                            }
                            frame "Aller à la pos. ref." {
                              n152 = call "MoveSinglePIMotor.vi"("System no."=w235, "Axes to move"=w231, "Go home"=w232) -> ("Position"=w234:dbl[], "error out"=w233:errorcluster)  [unwired: 15 in]
                            }
                          }
                          n153 = local write "Position Moteurs (PI) 2"(w198) -> ()
                          n154 = shared-variable "My Computer\\PSP Variables Lib.lvlib\\Position Moteurs PI 2 PSP"(w198) -> ()  [unwired: 1 in, 1 out]
                        }
                      }
                    }
                    frame #3 {
                      n155 = property on="Stop Mvt" class="Bool (strict)"("Value"=FALSE ("Stop Mvt")) -> ()  [unwired: 2 in, 2 out]
                    }
                  }
                }
              }
            }
            event "MVT-": Value Change {
              n156 = event-data() -> ()  [unwired: 1 in, 6 out]
              n157 = local read "Axe à déplacer (PI)"() -> (w237:T5)
              n158 = Less?(x=w237, y=4) -> (x < y?=w238:bool)
              n159 = case shown="False" w238 {
                tunnel: w237 -> [w245 w259]
                frame False {
                  n160 = local read "Axes \nConn. 2"() -> (w253:string[])
                  n161 = Subtract(x=w245, y=4) -> (x-y=w243:i32)
                  n162 = local read "error out \nPI Enceinte 2"() -> (w248:errorcluster)
                  n163 = local read "Déplacement"() -> (w250:dbl[])
                  n164 = local read "SafeMax 2"() -> (w241:dbl[])
                  n165 = local read "SafeMin 2"() -> (w240:dbl[])
                  n166 = Array Subset(array=w253, index=w243, length=1) -> (w251:string[])
                  n167 = control-ref of="Stop Mvt"() -> (w249:refnum<vi>)
                  n168 = call "MoveSinglePIMotor.vi"("System no."=2, "Axes to move"=w251, "Move"=w250, "SafeMax"=w241, "SafeMin"=w240, "error in"=w248, "Move relative (-)"=TRUE ("Move relative (+)"), "Stop refnum"=w249) -> ("Position"=w242:dbl[], "error out"=w247:errorcluster)  [unwired: 10 in]
                  n169 = local write "Position Moteurs (PI) 2"(w242) -> ()
                  n170 = local write "Position 2"(w242) -> ()
                  n171 = shared-variable "My Computer\\PSP Variables Lib.lvlib\\Position Moteurs PI 2 PSP"(w242) -> ()  [unwired: 1 in, 1 out]
                  n172 = flat-sequence {
                    tunnel: w247 -> [w256]
                    frame #0 {
                      n173 = local write "error out \nPI Enceinte 2"(w256) -> ()
                      n174 = local write "Stop Mvt"(FALSE ("Stop Mvt")) -> ()
                    }
                  }
                }
                frame True {
                  n175 = local read "Axes \nConn."() -> (w268:string[])
                  n176 = local read "error out \nPI Enceinte"() -> (w263:errorcluster)
                  n177 = local read "Déplacement"() -> (w265:dbl[])
                  n178 = local read "SafeMax 1"() -> (w258:dbl[])
                  n179 = local read "SafeMin 1"() -> (w257:dbl[])
                  n180 = Array Subset(array=w268, index=w259, length=1) -> (w266:string[])
                  n181 = control-ref of="Stop Mvt"() -> (w264:refnum<vi>)
                  n182 = call "MoveSinglePIMotor.vi"("System no."=1, "Axes to move"=w266, "Move"=w265, "SafeMax"=w258, "SafeMin"=w257, "error in"=w263, "Move relative (-)"=TRUE ("Move relative (+)"), "Stop refnum"=w264) -> ("Position"=w260:dbl[], "error out"=w262:errorcluster)  [unwired: 10 in]
                  n183 = local write "Position Moteurs (PI)"(w260) -> ()
                  n184 = shared-variable "My Computer\\PSP Variables Lib.lvlib\\Position Moteurs PI PSP"(w260) -> ()  [unwired: 1 in, 1 out]
                  n185 = flat-sequence {
                    tunnel: w262 -> [w271]
                    frame #0 {
                      n186 = local write "error out \nPI Enceinte"(w271) -> ()
                      n187 = local write "Stop Mvt"(FALSE ("Stop Mvt")) -> ()
                    }
                  }
                }
              }
            }
            event "MVT+": Value Change {
              n188 = event-data() -> ()  [unwired: 1 in, 6 out]
              n189 = local read "Axe à déplacer (PI)"() -> (w273:T5)
              n190 = Less?(x=w273, y=4) -> (x < y?=w272:bool)
              n191 = case shown="False" w272 {
                tunnel: w273 -> [w280 w302]
                frame False {
                  n192 = Subtract(x=w280, y=4) -> (x-y=w278:i32)
                  n193 = local read "Axes \nConn."() -> (w288:string[])
                  n194 = local read "error out \nPI Enceinte"() -> (w283:errorcluster)
                  n195 = local read "SafeMax 2"() -> (w276:dbl[])
                  n196 = local read "SafeMin 2"() -> (w275:dbl[])
                  n197 = Array Subset(array=w288, index=w278, length=1 ("longueur")) -> (w286:string[])
                  n198 = local read "Déplacement"() -> (w285:dbl[])
                  n199 = control-ref of="Stop Mvt"() -> (w284:refnum<vi>)
                  n200 = call "MoveSinglePIMotor.vi"("System no."=2, "Axes to move"=w286, "Move"=w285, "SafeMax"=w276, "SafeMin"=w275, "error in"=w283, "Move relative (+)"=TRUE, "Stop refnum"=w284) -> ("Position"=w277:dbl[], "error out"=w282:errorcluster)  [unwired: 10 in]
                  n201 = local write "Position Moteurs (PI) 2"(w277) -> ()
                  n202 = flat-sequence {
                    tunnel: w282 -> [w291]
                    frame #0 {
                      n203 = local write "error out \nPI Enceinte"(w291) -> ()
                      n204 = local write "Stop Mvt"(FALSE ("Stop Mvt")) -> ()
                    }
                  }
                  n205 = local write "Position 2"(w277) -> ()
                  n206 = shared-variable "My Computer\\PSP Variables Lib.lvlib\\Position Moteurs PI 2 PSP"(w277) -> ()  [unwired: 1 in, 1 out]
                }
                frame True {
                  n207 = local read "Axes \nConn."() -> (w303:string[])
                  n208 = Array Subset(array=w303, index=w302, length=1 ("longueur")) -> (w300:string[])
                  n209 = local read "Déplacement"() -> (w299:dbl[])
                  n210 = local read "SafeMax 1"() -> (w293:dbl[])
                  n211 = local read "SafeMin 1"() -> (w292:dbl[])
                  n212 = local read "error out \nPI Enceinte"() -> (w297:errorcluster)
                  n213 = control-ref of="Stop Mvt"() -> (w298:refnum<vi>)
                  n214 = call "MoveSinglePIMotor.vi"("System no."=1, "Axes to move"=w300, "Move"=w299, "SafeMax"=w293, "SafeMin"=w292, "error in"=w297, "Move relative (+)"=TRUE, "Stop refnum"=w298) -> ("Position"=w294:dbl[], "error out"=w296:errorcluster)  [unwired: 10 in]
                  n215 = local write "Position Moteurs (PI)"(w294) -> ()
                  n216 = local write "Position"(w294) -> ()
                  n217 = flat-sequence {
                    tunnel: w296 -> [w306]
                    frame #0 {
                      n218 = local write "error out \nPI Enceinte"(w306) -> ()
                      n219 = local write "Stop Mvt"(FALSE ("Stop Mvt")) -> ()
                    }
                  }
                  n220 = shared-variable "My Computer\\PSP Variables Lib.lvlib\\Position Moteurs PI PSP"(w294) -> ()  [unwired: 1 in, 1 out]
                }
              }
            }
            event "Set Ref (PI)": Value Change {
              n221 = event-data() -> ()  [unwired: 1 in, 6 out]
              n222 = property on="Axe (PI refs)" class="Enum (strict)"() -> ("Value"=w307:T5)  [unwired: 2 in, 2 out]
              n223 = case shown="\"Target Transverse\"..\"Mitu Obj Transverse\"" w307 {
                frame "Objective Focus".."<unassigned 1, 4>" {
                  n224 = local read "error out \nPI Enceinte"() -> (w308:errorcluster)
                  n225 = call "GetPos.vi"("System no."=1, "error in"=w308) -> ("Position"=w315:dbl[], "error out"=w311:errorcluster)  [unwired: 16 in]
                  n226 = local write "error out \nPI Enceinte"(w311) -> ()
                  n227 = local read "Axe (PI refs)"() -> (w310:T5)
                  n228 = local read "Référence"() -> (w313:T6)
                  n229 = local read "Positions de référence"() -> (w314:dbl[][])
                  n230 = Index Array(array=w315, index=w310) -> (element=w309:dbl)
                  n231 = Replace Array Subset(array=w314, new element=w309, index (row)=w310, index (col)=w313) -> (w312:dbl[][])
                  n232 = local write "Positions de référence"(w312) -> ()
                }
                frame "Target Transverse".."Mitu Obj Transverse" {
                  n233 = local read "error out \nPI Enceinte 2"() -> (w324:errorcluster)
                  n234 = call "GetPos.vi"("System no."=2, "error in"=w324) -> ("Position"=w328:dbl[], "error out"=w326:errorcluster)  [unwired: 16 in]
                  n235 = local write "error out \nPI Enceinte 2"(w326) -> ()
                  n236 = local read "Axe (PI refs)"() -> (w322:T5)
                  n237 = Subtract(x=w322, y=4) -> (x-y=w317:i32)
                  n238 = local read "Référence"() -> (w319:T6)
                  n239 = local read "Positions de référence 2"() -> (w327:dbl[][])
                  n240 = Index Array(array=w328, index=w317) -> (element=w325:dbl)
                  n241 = To Long Integer(number=w319) -> (32bit integer=w318:i32)
                  n242 = To Long Integer(number=w317) -> (32bit integer=w320:i32)
                  n243 = Replace Array Subset(array=w327, new element=w325, index (row)=w320, index (col)=w318) -> (w321:dbl[][])
                  n244 = property on="Positions de référence 2" class="Arr (strict)"("Value"=w321) -> ()  [unwired: 2 in, 2 out]
                }
              }
            }
            event "Go to Ref (PI)": Value Change {
              # "UNFINISHED!!"
              n245 = event-data() -> ()  [unwired: 1 in, 6 out]
              n246 = local read "Axe (PI refs)"() -> (w332:T5)
              n247 = Less?(x=w332, y=4) -> (x < y?=w330:bool)
              n248 = case shown="True" w330 {
                frame False {
                  n249 = local read "Positions de référence 2"() -> (w350:dbl[][])
                  n250 = local read "Axe (PI refs)"() -> (w337:T5)
                  n251 = Reshape Array(w350, 16 ("dimension size")) -> (w348:dbl[])
                  n252 = local read "Référence"() -> (w344:T6)
                  n253 = Subtract(x=w337, y=4) -> (x-y=w336:i32)
                  n254 = local read "Axes \nConn. 2"() -> (w354:string[])
                  n255 = Multiply(x=w336, y=4) -> (x*y=w345:i32)
                  n256 = Array Subset(array=w354, length=1) -> (w353:string[])  [unwired: 1 in]
                  n257 = Add(x=w345, y=w344) -> (x+y=w343:i32)
                  n258 = control-ref of="Stop Mvt"() -> (w341:refnum<vi>)
                  n259 = Array Subset(array=w348, index=w343, length=1) -> (w347:dbl[])
                  n260 = local read "SafeMax 2"() -> (w334:dbl[])
                  n261 = local read "SafeMin 2"() -> (w333:dbl[])
                  n262 = local read "error out \nPI Enceinte"() -> (w339:errorcluster)
                  n263 = call "MoveSinglePIMotor.vi"("System no."=2, "Axes to move"=w353, "Move"=w347, "SafeMax"=w334, "SafeMin"=w333, "error in"=w339, "Move absolute"=TRUE, "Stop refnum"=w341) -> ("Position"=w335:dbl[], "error out"=w351:errorcluster)  [unwired: 10 in]
                  n264 = local write "Position Moteurs (PI) 2"(w335) -> ()
                  n265 = local write "Position 2"(w335) -> ()
                  n266 = shared-variable "My Computer\\PSP Variables Lib.lvlib\\Position Moteurs PI 2 PSP"(w335) -> ()  [unwired: 1 in, 1 out]
                  n267 = flat-sequence {
                    tunnel: w351 -> [w357]
                    frame #0 {
                      n268 = local write "error out \nPI Enceinte"(w357) -> ()
                      n269 = local write "Stop Mvt"(FALSE ("Stop Mvt")) -> ()
                    }
                  }
                }
                frame True {
                  n270 = local read "Positions de référence"() -> (w374:dbl[][])
                  n271 = local read "Axe (PI refs)"() -> (w362:T5)
                  n272 = Reshape Array(w374, 16 ("dimension size")) -> (w372:dbl[])
                  n273 = local read "Référence"() -> (w368:T6)
                  n274 = local read "Axe (PI refs)"() -> (w360:T5)
                  n275 = local read "Axes \nConn."() -> (w378:string[])
                  n276 = Multiply(x=w362, y=4) -> (x*y=w369:i32)
                  n277 = Array Subset(array=w378, index=w360, length=1) -> (w377:string[])
                  n278 = Add(x=w369, y=w368) -> (x+y=w367:i32)
                  n279 = control-ref of="Stop Mvt"() -> (w365:refnum<vi>)
                  n280 = Array Subset(array=w372, index=w367, length=1) -> (w371:dbl[])
                  n281 = local read "SafeMax 1"() -> (w359:dbl[])
                  n282 = local read "SafeMin 1"() -> (w358:dbl[])
                  n283 = local read "error out \nPI Enceinte"() -> (w363:errorcluster)
                  n284 = call "MoveSinglePIMotor.vi"("System no."=1, "Axes to move"=w377, "Move"=w371, "SafeMax"=w359, "SafeMin"=w358, "error in"=w363, "Move absolute"=TRUE, "Stop refnum"=w365) -> ("Position"=w361:dbl[], "error out"=w375:errorcluster)  [unwired: 10 in]
                  n285 = local write "Position Moteurs (PI)"(w361) -> ()
                  n286 = local write "Position"(w361) -> ()
                  n287 = flat-sequence {
                    tunnel: w375 -> [w381]
                    frame #0 {
                      n288 = local write "error out \nPI Enceinte"(w381) -> ()
                      n289 = local write "Stop Mvt"(FALSE ("Stop Mvt")) -> ()
                    }
                  }
                  n290 = shared-variable "My Computer\\PSP Variables Lib.lvlib\\Position Moteurs PI PSP"(w361) -> ()  [unwired: 1 in, 1 out]
                }
              }
            }
            event "Save": Value Change {
              n291 = event-data() -> ()  [unwired: 1 in, 6 out]
              n292 = local read "Nom Fichier Refs PI"() -> (w389:string)
              n293 = Current VI's Path() -> (path=w393:path)
              n294 = Strip Path(path=w393) -> (stripped path=w392:path)  [unwired: 1 out]
              n295 = Path To String(path=w392) -> (string=w391:string)
              n296 = local read "Positions de référence 2"() -> (w385:dbl[][])
              n297 = local read "Positions de référence"() -> (w383:dbl[][])
              n298 = Concatenate Strings(w391, "\\Moteurs PI\\PI Refs\\", w389, ".dat" ("string")) -> (w387:string)
              n299 = String To Path(string=w387) -> (path=w386:path)
              n300 = Insert Into Array(array=w385, index (row)=0, new element=w383) -> (w382:dbl[][])  [unwired: 1 in]
              n301 = call "SaveRefs.vi"("Références à charger"=w382, "file path (use dialog)"=w386) -> ("error out"=w394:errorcluster)  [unwired: 8 in]
              n302 = local write "error out\nLabview functions"(w394) -> ()
            }
            event "stop": Value Change {
              w395 = TRUE
              n303 = event-data() -> ()  [unwired: 1 in, 6 out]
            }
            event "Commande onglets": Value Change {
              n304 = event-data() -> ("OldVal"=w398:T2)  [unwired: 1 in, 5 out]
              n305 = Equal?(x=w398, y=T2."Mouvement moteurs enceinte (PI)" ("Commande onglets")) -> (x = y?=w396:bool)
            }
            event "Load": Value Change {
              n306 = event-data() -> ()  [unwired: 1 in, 6 out]
              n307 = call "LoadRefs.vi"("Number of axes"=8, "Number of refs"=4) -> ("Références à enregistrer"=w401:dbl[][], "error out"=w409:errorcluster)  [unwired: 7 in]
              n308 = Array Subset(array=w401, index (row)=4 ("index"), length (col)=4 ("length")) -> (w407:dbl[][])  [unwired: 2 in]
              n309 = Array Subset(array=w401, index (row)=0 ("index"), length (row)=4 ("length"), length (col)=4 ("length")) -> (w408:dbl[][])  [unwired: 1 in]
              n310 = local write "error out\nLabview functions"(w409) -> ()
              n311 = local write "Positions de référence"(w408) -> ()
              n312 = local write "Positions de référence 2"(w407) -> ()
            }
          }
        }
      }
      frame "Mouvement PilMot" {
        n313 = while {
          tunnel: [w412] -> w410
          stop <- w411 stop-if-true
          n314 = event shown="[9] \"Load Ref PilMot\": Value Change" {
            selector: _ -> [_ _ _ _ _ _ _ _ _ _ _]
            dyn-events: _ -> [_ _ _ _ _ _ _ _ _ _ _]
            timeout: _ -> [_ _ _ _ _ _ _ _ _ _ _]
            tunnel: [w413 _ _ _ w458 _ _ _ _ _ _] -> w411
            tunnel: [_ _ _ _ w458 _ _ _ _ _ _] -> w412
            event "Commande onglets": Value Change {
              # "Stops event structure"
              n315 = event-data() -> ("OldVal"=w415:T2)  [unwired: 1 in, 5 out]
              n316 = Equal?(x=w415, y=T2."Mouvement PilMot" ("Commande onglets")) -> (x = y?=w413:bool)
            }
            event "Aller à CàA": Value Change {
              n317 = event-data() -> ()  [unwired: 1 in, 6 out]
              n318 = local read "Axes à déplacer \n(PilMot)"() -> (w422:bool[])
              n319 = local read "Cotes à atteindre"() -> (w419:dbl[])
              n320 = local read "Coeff µm/pas"() -> (w417:dbl[])
              n321 = local read "Vitesses"() -> (w421:i32[])
              n322 = local read "Mouvement Rel/Abs"() -> (w420:u16)
              n323 = call "ConvertStepsmm.vi"("Conversion: T: pas->mm\n                      F: mm->pas"=FALSE ("Conversion: T: pas->mm\n                      F: mm->pas"), "Input en mm"=w419, "Facteur de conversion\n en µm/pas"=w417) -> ("output en pas"=w418:i32[])  [unwired: 7 in, 1 out]
              n324 = for {
                tunnel: w422 -> [w427] mode=indexing
                tunnel: w421 -> [w426] mode=indexing
                tunnel: w420 -> [w425]
                tunnel: w418 -> [w424] mode=indexing
                i -> [w428]
                n325 = case shown="True" w427 {
                  tunnel: w428 -> [_ w437]
                  tunnel: w426 -> [_ w436]
                  tunnel: w425 -> [_ w435]
                  tunnel: w424 -> [_ w434]
                  frame False {
                  }
                  frame True {
                    w439 = T10 2 items=["Mouvement Simple"=1, "Aller vers Cote"=2] ("Type de mouvement")
                    # "Va vers cote"
                    n326 = property on="Envoi cmde PilMot?" class="Bool (strict)"("Value"=TRUE ("Sending PilMot command")) -> (error out=w432:errorcluster)  [unwired: 2 in, 1 out]
                    n327 = Increment(x=w437) -> (x+1=w442:i32)
                    n328 = local read "Adresse du PilMOT"() -> (w441:string)
                    n329 = call "FetchAxisSharedVars.vi"("error in (no error)"=w432, "Numéro d'Axe"=w442, "PilMOT Address"=w441) -> ("error out"=w440:errorcluster, "Sortie Variables d'Axes"=w438:T11)  [unwired: 7 in]
                    n330 = call "MovePilMot.vi"("Variables d'Axes"=w438, "Cote à atteindre"=w434, "Vitesse"=w436, "error in (no error)"=w440, "Type de mouvement"=w439, "Mouvement Absolu/Relatif"=w435) -> ("error out"=w430:errorcluster)  [unwired: 9 in]
                    n331 = property on="Envoi cmde PilMot?" class="Bool (strict)"(error in=w430, "Value"=FALSE ("Sending PilMot command")) -> (error out=w429:errorcluster)  [unwired: 1 in, 1 out]
                    n332 = local write "error out\nesbim"(w429) -> ()
                  }
                }
                n333 = Wait Until Next ms Multiple(millisecond multiple=u32 200 ("n millisecondes")) -> ()  [unwired: 1 out]
              }
            }
            event "Déplacement +": Value Change {
              w454 = T10 1 items=["Mouvement Simple"=1, "Aller vers Cote"=2] ("Type de mouvement")
              n334 = event-data() -> ()  [unwired: 1 in, 6 out]
              n335 = property on="Envoi cmde PilMot?" class="Bool (strict)"("Value"=TRUE ("Sending PilMot command")) -> (error out=w445:errorcluster)  [unwired: 2 in, 1 out]
              n336 = local read "Adresse du PilMOT"() -> (w450:string)
              n337 = local read "Axe à déplacer"() -> (w451:u16)
              n338 = call "FetchAxisSharedVars.vi"("error in (no error)"=w445, "Numéro d'Axe"=w451, "PilMOT Address"=w450) -> ("error out"=w453:errorcluster, "Sortie Variables d'Axes"=w452:T11)  [unwired: 7 in]
              n339 = call "MovePilMot.vi"("Ordre UC"=u16 16, "Variables d'Axes"=w452, "error in (no error)"=w453, "Type de mouvement"=w454, "Ordre Bloc"=u16 0 ("cas faux")) -> ("error out"=w444:errorcluster)  [unwired: 10 in]
              n340 = property on="Envoi cmde PilMot?" class="Bool (strict)"(error in=w444, "Value"=FALSE ("Sending PilMot command")) -> (error out=w443:errorcluster)  [unwired: 1 in, 1 out]
              n341 = local write "error out\nesbim"(w443) -> ()
            }
            event "STOP MOTEURS!!": Value Change {
              n342 = event-data() -> ()  [unwired: 1 in, 6 out]
              n343 = stacked-sequence {
                frame #0 {
                  n344 = property on="Envoi cmde PilMot?" class="Bool (strict)"("Value"=TRUE ("Sending PilMot command")) -> ()  [unwired: 2 in, 2 out]
                }
                frame #1 {
                  n345 = call "Arret Urgence.vi"() -> ("error out"=w456:errorcluster)  [unwired: 11 in]
                  n346 = local write "error out\nesbim"(w456) -> ()
                }
                frame #2 {
                  n347 = property on="Envoi cmde PilMot?" class="Bool (strict)"("Value"=FALSE ("Sending PilMot command")) -> ()  [unwired: 2 in, 2 out]
                }
              }
            }
            event "stop": Value Change {
              w458 = TRUE
              n348 = event-data() -> ()  [unwired: 1 in, 6 out]
              n349 = property on="Envoi cmde PilMot?" class="Bool (strict)"("Value"=TRUE ("Sending PilMot command")) -> (error out=w462:errorcluster)  [unwired: 2 in, 1 out]
              n350 = flat-sequence {
                tunnel: [w464] -> w460
                tunnel: w462 -> [_]
                frame #0 {
                  n351 = call "Arret Urgence.vi"() -> ("error out"=w464:errorcluster)  [unwired: 11 in]
                }
              }
              n352 = property on="Envoi cmde PilMot?" class="Bool (strict)"(error in=w460, "Value"=FALSE ("Sending PilMot command")) -> (error out=w459:errorcluster)  [unwired: 1 in, 1 out]
              n353 = local write "error out\nesbim"(w459) -> ()
            }
            event "Déplacement -": Value Change {
              w476 = T10 1 items=["Mouvement Simple"=1, "Aller vers Cote"=2] ("Type de mouvement")
              # "Mouvement simple:\nAvance (16)\nRecule (32)\nStop (8)\nOrigine (16)"
              n354 = event-data() -> ()  [unwired: 1 in, 6 out]
              n355 = property on="Envoi cmde PilMot?" class="Bool (strict)"("Value"=TRUE ("Sending PilMot command")) -> (error out=w465:errorcluster)  [unwired: 2 in, 1 out]
              n356 = local read "Adresse du PilMOT"() -> (w472:string)
              n357 = local read "Axe à déplacer"() -> (w473:u16)
              n358 = call "FetchAxisSharedVars.vi"("error in (no error)"=w465, "Numéro d'Axe"=w473, "PilMOT Address"=w472) -> ("error out"=w475:errorcluster, "Sortie Variables d'Axes"=w474:T11)  [unwired: 7 in]
              n359 = call "MovePilMot.vi"("Ordre UC"=u16 32 ("cas vrai"), "Variables d'Axes"=w474, "error in (no error)"=w475, "Type de mouvement"=w476, "Ordre Bloc"=u16 0 ("cas faux")) -> ("error out"=w467:errorcluster)  [unwired: 10 in]
              n360 = property on="Envoi cmde PilMot?" class="Bool (strict)"(error in=w467, "Value"=FALSE ("Sending PilMot command")) -> (error out=w466:errorcluster)  [unwired: 1 in, 1 out]
              n361 = local write "error out\nesbim"(w466) -> ()
            }
            event "Set Ref (PilMot)": Value Change {
              n362 = event-data() -> ()  [unwired: 1 in, 6 out]
              n363 = property on="Référence PilMot" class="Enum (strict)"() -> ("Value"=w483:T6)  [unwired: 2 in, 2 out]
              n364 = property on="Axe à déplacer PilMot" class="Ring (strict)"() -> ("Value"=w481:u16)  [unwired: 2 in, 2 out]
              n365 = case shown="6" w481 {
                tunnel: [0 1 2 3 4 5] -> w484
                tunnel: w483 -> [w491 w493 w500 w507 w514 w521]
                tunnel: [w491 w493 w500 w507 w514 w521] -> w482
                tunnel: [w488 w494 w501 w508 w515 w522] -> w478
                frame 1, Default {
                  n366 = shared-variable "My Computer\\OPC.lvlib\\Axe1_PositionTheorique"() -> (w487:i32)  [unwired: 1 in, 1 out]
                  n367 = property on="Coeff µm/pas" class="Arr (strict)"() -> ("Value"=w490:dbl[])  [unwired: 2 in, 2 out]
                  n368 = Index Array(array=w490, index=0) -> (element=w486:dbl)
                  n369 = Multiply(x=w487, y=w486) -> (x*y=w488:dbl)
                }
                frame 2 {
                  n370 = shared-variable "My Computer\\OPC.lvlib\\Axe2_PositionTheorique"() -> (w495:i32)  [unwired: 1 in, 1 out]
                  n371 = property on="Coeff µm/pas" class="Arr (strict)"() -> ("Value"=w498:dbl[])  [unwired: 2 in, 2 out]
                  n372 = Index Array(array=w498, index=1) -> (element=w496:dbl)
                  n373 = Multiply(x=w495, y=w496) -> (x*y=w494:dbl)
                }
                frame 3 {
                  n374 = shared-variable "My Computer\\OPC.lvlib\\Axe3_PositionTheorique"() -> (w502:i32)  [unwired: 1 in, 1 out]
                  n375 = property on="Coeff µm/pas" class="Arr (strict)"() -> ("Value"=w505:dbl[])  [unwired: 2 in, 2 out]
                  n376 = Index Array(array=w505, index=2) -> (element=w503:dbl)
                  n377 = Multiply(x=w502, y=w503) -> (x*y=w501:dbl)
                }
                frame 4 {
                  n378 = shared-variable "My Computer\\OPC.lvlib\\Axe4_PositionTheorique"() -> (w509:i32)  [unwired: 1 in, 1 out]
                  n379 = property on="Coeff µm/pas" class="Arr (strict)"() -> ("Value"=w512:dbl[])  [unwired: 2 in, 2 out]
                  n380 = Index Array(array=w512, index=3) -> (element=w510:dbl)
                  n381 = Multiply(x=w509, y=w510) -> (x*y=w508:dbl)
                }
                frame 5 {
                  n382 = shared-variable "My Computer\\OPC.lvlib\\Axe5_PositionTheorique"() -> (w516:i32)  [unwired: 1 in, 1 out]
                  n383 = property on="Coeff µm/pas" class="Arr (strict)"() -> ("Value"=w519:dbl[])  [unwired: 2 in, 2 out]
                  n384 = Index Array(array=w519, index=4) -> (element=w517:dbl)
                  n385 = Multiply(x=w516, y=w517) -> (x*y=w515:dbl)
                }
                frame 6 {
                  n386 = shared-variable "My Computer\\OPC.lvlib\\Axe6_PositionTheorique"() -> (w523:i32)  [unwired: 1 in, 1 out]
                  n387 = property on="Coeff µm/pas" class="Arr (strict)"() -> ("Value"=w526:dbl[])  [unwired: 2 in, 2 out]
                  n388 = Index Array(array=w526, index=5) -> (element=w524:dbl)
                  n389 = Multiply(x=w523, y=w524) -> (x*y=w522:dbl)
                }
              }
              n390 = property on="Positions de référence PilMot" class="Arr (strict)"() -> ("Value"=w485:dbl[][])  [unwired: 2 in, 2 out]
              n391 = Divide(x=w478, y=1000.0) -> (x/y=w479:dbl)
              n392 = Replace Array Subset(array=w485, new element=w479, index (row)=w484, index (col)=w482) -> (w480:dbl[][])
              n393 = property on="Positions de référence PilMot" class="Arr (strict)"("Value"=w480) -> ()  [unwired: 2 in, 2 out]
            }
            event "Go to Ref (PilMot)": Value Change {
              w538 = u16 0 items=["Mouvement Relatif"=1, "Mouvement Absolu"=0] ("Mouvement Absolu/Relatif")
              w539 = T10 2 items=["Mouvement Simple"=1, "Aller vers Cote"=2] ("Type de mouvement")
              n394 = event-data() -> ()  [unwired: 1 in, 6 out]
              n395 = local read "Positions de référence PilMot"() -> (w546:dbl[][])
              n396 = local read "Axe à déplacer PilMot"() -> (w549:T8)
              n397 = local read "Référence PilMot"() -> (w545:T6)
              n398 = local read "Coeff µm/pas"() -> (w550:dbl[])
              n399 = Decrement(x=w549) -> (x-1=w544:T8)
              n400 = Index Array(array=w550, index=w544) -> (element=w548:dbl)
              n401 = Index Array(array=w546, index (row)=w544, index (col)=w545) -> (element=w543:dbl)
              n402 = Build Array(w548) -> (w547:dbl[])
              n403 = local read "Axe à déplacer PilMot"() -> (w540:T8)
              n404 = local read "Adresse du PilMOT"() -> (w541:string)
              n405 = Build Array(w543) -> (w542:dbl[])
              n406 = call "ConvertStepsmm.vi"("Conversion: T: pas->mm\n                      F: mm->pas"=FALSE ("Conversion: T: pas->mm\n                      F: mm->pas"), "Input en mm"=w542, "Facteur de conversion\n en µm/pas"=w547) -> ("output en pas"=w536:i32[])  [unwired: 7 in, 1 out]
              n407 = property on="Envoi cmde PilMot?" class="Bool (strict)"("Value"=TRUE ("Sending PilMot command")) -> (error out=w532:errorcluster)  [unwired: 2 in, 1 out]
              n408 = Index Array(array=w536, index=0) -> (element=w534:i32)
              n409 = call "FetchAxisSharedVars.vi"("error in (no error)"=w532, "Numéro d'Axe"=w540, "PilMOT Address"=w541) -> ("error out"=w531:errorcluster, "Sortie Variables d'Axes"=w537:T11)  [unwired: 7 in]
              n410 = call "MovePilMot.vi"("Variables d'Axes"=w537, "Cote à atteindre"=w534, "error in (no error)"=w531, "Type de mouvement"=w539, "Mouvement Absolu/Relatif"=w538) -> ("error out"=w528:errorcluster)  [unwired: 10 in]
              n411 = property on="Envoi cmde PilMot?" class="Bool (strict)"(error in=w528, "Value"=FALSE ("Sending PilMot command")) -> (error out=w529:errorcluster)  [unwired: 1 in, 1 out]
              n412 = local write "error out\nesbim"(w529) -> ()
            }
            event "Save Ref PilMot": Value Change {
              n413 = event-data() -> ()  [unwired: 1 in, 6 out]
              n414 = local read "Nom Fichier Refs PilMOT"() -> (w553:string)
              n415 = Current VI's Path() -> (path=w560:path)
              n416 = Strip Path(path=w560) -> (stripped path=w559:path)  [unwired: 1 out]
              n417 = Path To String(path=w559) -> (string=w558:string)
              n418 = Concatenate Strings(w558, "\\PilMOT\\RefsMoteurs\\", w553, ".dat" ("string")) -> (w555:string)
              n419 = local read "Positions de référence PilMot"() -> (w552:dbl[][])
              n420 = String To Path(string=w555) -> (path=w554:path)
              n421 = call "SaveRefs.vi"("Références à charger"=w552, "file path (use dialog)"=w554) -> ("error out"=w561:errorcluster)  [unwired: 8 in]
              n422 = local write "error out\nLabview functions"(w561) -> ()
            }
            event "Load Ref PilMot": Value Change {
              n423 = event-data() -> ()  [unwired: 1 in, 6 out]
              n424 = call "LoadRefs.vi"("Number of axes"=6, "Number of refs"=4) -> ("Références à enregistrer"=w564:dbl[][])  [unwired: 7 in, 1 out]
              n425 = property on="Positions de référence PilMot" class="Arr (strict)"("Value"=w564) -> ()  [unwired: 2 in, 2 out]
            }
            event "Origine": Value Change {
              w576 = T10 1 items=["Mouvement Simple"=1, "Aller vers Cote"=2] ("Type de mouvement")
              # "Mouvement simple:\nAvance (16)\nRecule (32)\nStop (8)\nOrigine (16)"
              n426 = event-data() -> ()  [unwired: 1 in, 6 out]
              n427 = property on="Envoi cmde PilMot?" class="Bool (strict)"("Value"=TRUE ("Sending PilMot command")) -> (error out=w568:errorcluster)  [unwired: 2 in, 1 out]
              n428 = local read "Adresse du PilMOT"() -> (w572:string)
              n429 = local read "Axe à déplacer"() -> (w573:u16)
              n430 = call "FetchAxisSharedVars.vi"("error in (no error)"=w568, "Numéro d'Axe"=w573, "PilMOT Address"=w572) -> ("error out"=w575:errorcluster, "Sortie Variables d'Axes"=w574:T11)  [unwired: 7 in]
              n431 = call "MovePilMot.vi"("Ordre UC"=u16 2, "Variables d'Axes"=w574, "error in (no error)"=w575, "Type de mouvement"=w576, "Ordre Bloc"=u16 16) -> ("error out"=w566:errorcluster)  [unwired: 10 in]
              n432 = property on="Envoi cmde PilMot?" class="Bool (strict)"(error in=w566, "Value"=FALSE ("Sending PilMot command")) -> (error out=w565:errorcluster)  [unwired: 1 in, 1 out]
              n433 = local write "error out\nesbim"(w565) -> ()
            }
          }
        }
      }
      frame "Mouvement Ligne à retard (PI)" {
        n434 = stacked-sequence {
          tunnel: [_ w605] -> w577
          frame #0 {
            # "Actualise la valeur du zéro"
            n435 = local read "Fichier zéro ligne à retard"() -> (w581:path)
            n436 = Open/Create/Replace File(file path (use dialog)=w581, error in=errorcluster {"status"=FALSE, "code"=0, "source"=""}, operation (0:open)=T9."open") -> (error out=w580:errorcluster)  [unwired: 3 in, 2 out]
            n437 = Unbundle By Name(w580) -> ("code"=w583:i32, "status"=w582:bool)
            n438 = Equal?(x=7 ("code"), y=w583) -> (x = y?=w585:bool)
            n439 = case shown="True" w585 {
              tunnel: w582 -> [w590 _]
              tunnel: w581 -> [w588 w596]
              tunnel: w580 -> [w589 _]
              tunnel: [w587 w599] -> w579
              frame False {
                n440 = case shown="False" w590 {
                  tunnel: w589 -> [w593 w594]
                  tunnel: w588 -> [w592 _]
                  tunnel: [w591 _] -> w587
                  frame False {
                    n441 = Scan From String(w592, w593) -> (output 1=w591:dbl)  [unwired: 2 in, 2 out]
                    n442 = global write "Zero.vi" "Zero"(w591) -> ()
                  }
                  frame True {
                    n443 = local write "error out\nLabview functions"(w594) -> ()
                  }
                }
              }
              frame True {
                w599 = 0.0 ("input 1")
                n444 = Open/Create/Replace File(file path (use dialog)=w596, error in=errorcluster {"status"=FALSE, "code"=0, "source"=""}, operation (0:open)=T9."replace or create", access (0:read/write)=enum16{"read/write", "read-only", "write-only"}."read/write") -> (refnum out=w603:refnum<file>, error out=w602:errorcluster)  [unwired: 2 in, 1 out]
                n445 = Format Into String(initial string=w603, error in=w602, w599) -> (resulting string=w600:refnum<file>, error out=w601:errorcluster)  [unwired: 1 in]
                n446 = Close File(refnum=w600, error in=w601) -> (error out=w598:errorcluster)  [unwired: 1 out]
                n447 = local write "error out\nLabview functions"(w598) -> ()
              }
            }
            n448 = local write "Current zero position"(w579) -> ()
          }
          frame #1 {
            n449 = while {
              tunnel: [w606] -> w605
              stop <- w607 stop-if-true
              n450 = event shown="[4] \"JOG + delay\": Value Change" {
                selector: _ -> [_ _ _ _ _ _ _ _ _ _ _ _ _ _]
                dyn-events: _ -> [_ _ _ _ _ _ _ _ _ _ _ _ _ _]
                timeout: _ -> [_ _ _ _ _ _ _ _ _ _ _ _ _ _]
                tunnel: [w608 FALSE FALSE FALSE FALSE FALSE FALSE FALSE FALSE FALSE FALSE FALSE FALSE w883] -> w607
                tunnel: [_ _ _ _ _ _ _ _ _ _ _ _ _ w883] -> w606
                event "Commande onglets": Value Change {
                  n451 = event-data() -> ("OldVal"=w610:T2)  [unwired: 1 in, 5 out]
                  n452 = Equal?(x=w610, y=T2."Mouvement Ligne à retard (PI)" ("Commande onglets")) -> (x = y?=w608:bool)
                }
                event "Query Pos.": Value Change {
                  n453 = event-data() -> ()  [unwired: 1 in, 6 out]
                  n454 = local read "error out \nligne à retard"() -> (w614:errorcluster)
                  n455 = local read "Conn. \nAxes"() -> (w615:string[])
                  n456 = call "POS?.vi"("System no."=2, "Axes to query"=w615, "error in"=w614) -> ("Position"=w612:dbl[])  [unwired: 15 in, 1 out]
                  n457 = Index Array(array=w612) -> (element=w613:dbl)  [unwired: 1 in]
                  n458 = local write "Position de la ligne à retard"(w613) -> ()
                  n459 = local write "Position ligne à retard"(w612) -> ()
                }
                event "CLR ERR LàR": Value Change {
                  n460 = event-data() -> ()  [unwired: 1 in, 6 out]
                  n461 = stacked-sequence {
                    seq-local: [_ w621 _] -> [_ _ w627]
                    frame #0 {
                      n462 = local write "Ligne à retard prête?"(FALSE ("Ligne à retard prête?")) -> ()
                    }
                    frame #1 {
                      w622 = u16 2 items=["RS232", "RS232 DaisyChain", "USB", "USB_DaisyChain"] ("Interface")
                      n463 = call "Mercury_GCS_Configuration_Setup.vi"("System no."=2, "Interface"=w622, "error in"=errorcluster {"status"=FALSE, "code"=0, "source"=""}, "Switch servo on?"=TRUE) -> ("Position"=w620:dbl[], "error out"=w621:errorcluster)  [unwired: 9 in, 5 out]
                      n464 = Index Array(array=w620) -> (element=w619:dbl)  [unwired: 1 in]
                      n465 = local write "Position ligne à retard"(w620) -> ()
                      n466 = local write "Position de la ligne à retard"(w619) -> ()
                    }
                    frame #2 {
                      n467 = Unbundle By Name(w627) -> ("status"=w626:bool)
                      n468 = case shown="False" w626 {
                        frame False {
                          n469 = local write "Ligne à retard prête?"(TRUE ("Ligne à retard prête?")) -> ()
                        }
                        frame True {
                          n470 = local write "Ligne à retard prête?"(FALSE ("Ligne à retard prête?")) -> ()
                        }
                      }
                    }
                  }
                }
                event "JOG + position": Value Change {
                  w640 = 2 ("System no.")
                  n471 = event-data() -> ()  [unwired: 1 in, 6 out]
                  n472 = local read "error out \nligne à retard"() -> (w634:errorcluster)
                  n473 = local read "Position de la ligne à retard"() -> (w642:dbl)
                  n474 = flat-sequence {
                    tunnel: w634 -> [w644]
                    tunnel: [w644] -> w633
                    frame #0 {
                      n475 = property on="Ligne à retard prête?" class="Bool (strict)"("Value"=FALSE ("Ligne à retard prête?")) -> ()  [unwired: 2 in, 2 out]
                    }
                  }
                  n476 = local read "Step Size (mm)"() -> (w643:dbl)
                  n477 = local read "Conn. \nAxes"() -> (w639:string[])
                  n478 = Add(x=w643, y=w642) -> (x+y=w641:dbl)
                  n479 = control-ref of="Stop here"() -> (w631:refnum<vi>)
                  n480 = Build Array(w641) -> (w638:dbl[])
                  n481 = call "MoveSinglePIMotor_Mercury.vi"("System no."=w640, "Axes to move"=w639, 3:"Move"=w638, "error in"=w633, 11:"Move"=TRUE ("Move"), "Stop refnum"=w631) -> ("error out"=w637:errorcluster)  [unwired: 12 in, 1 out]
                  n482 = Unbundle By Name(w637) -> ("status"=w636:bool)
                  n483 = case shown="False" w636 {
                    tunnel: w640 -> [w650 w660]
                    tunnel: [w647 w658] -> w632
                    tunnel: w639 -> [w649 _]
                    tunnel: w637 -> [w648 w656]
                    frame False {
                      n484 = call "POS?.vi"("System no."=w650, "Axes to query"=w649, "error in"=w648) -> ("Position"=w646:dbl[], "error out"=w647:errorcluster)  [unwired: 15 in]
                      n485 = local write "Position ligne à retard"(w646) -> ()
                      n486 = Index Array(array=w646) -> (element=w653:dbl)  [unwired: 1 in]
                      n487 = local write "Position de la ligne à retard"(w653) -> ()
                      n488 = property on="Stop here" class="Bool (strict)"("Value"=FALSE ("Stop here")) -> ()  [unwired: 2 in, 2 out]
                      n489 = property on="Ligne à retard prête?" class="Bool (strict)"("Value"=TRUE ("Ligne à retard prête?")) -> ()  [unwired: 2 in, 2 out]
                    }
                    frame True {
                      n490 = call "ERR?.vi"("System no."=w660, "error in"=w656) -> ("error out"=w659:errorcluster)  [unwired: 16 in, 1 out]
                      n491 = call "GCSTranslateError.vi"("error in"=w659) -> ("Error Description"=w657:string, "error out"=w658:errorcluster)  [unwired: 16 in, 1 out]
                      n492 = property on="Stop here" class="Bool (strict)"("Value"=FALSE ("Stop here")) -> ()  [unwired: 2 in, 2 out]
                      n493 = local write "Error Description (delay line)"(w657) -> ()
                      n494 = property on="Ligne à retard prête?" class="Bool (strict)"("Value"=FALSE ("Ligne à retard prête?")) -> ()  [unwired: 2 in, 2 out]
                    }
                  }
                  n495 = local write "error out \nligne à retard"(w632) -> ()
                }
                event "JOG + delay": Value Change {
                  w678 = 2 ("System no.")
                  # "Division par 2 à cause\nde l'aller-retour sur la \nligne à retard"
                  n496 = event-data() -> ()  [unwired: 1 in, 6 out]
                  n497 = local read "Step Size (ps)"() -> (w680:dbl)
                  n498 = local read "error out \nligne à retard"() -> (w666:errorcluster)
                  n499 = Divide(x=w680, y=2.0) -> (x/y=w664:dbl)
                  n500 = local read "Position de la ligne à retard"() -> (w671:dbl)
                  n501 = Build Array(w664) -> (w679:dbl[])
                  n502 = call "SpaceTimeConversion.vi"("Conversion Type: T : Distance to Time\n                             F : Time to Distance"=FALSE ("Conversion Type: T : Distance to Time\n                             F : Time to Distance"), "Time IN (ps)"=w679, "Zero Position"=0.0) -> ("Time OUT (ps) / Distance OUT (mm)"=w673:dbl[])  [unwired: 1 in]
                  n503 = flat-sequence {
                    tunnel: w666 -> [w682]
                    tunnel: [w682] -> w665
                    frame #0 {
                      n504 = local write "Ligne à retard prête?"(FALSE ("Ligne à retard prête?")) -> ()
                    }
                  }
                  n505 = Index Array(array=w673) -> (element=w672:dbl)  [unwired: 1 in]
                  n506 = local read "Conn. \nAxes"() -> (w662:string[])
                  n507 = Add(x=w672, y=w671) -> (x+y=w670:dbl)
                  n508 = Build Array(w670) -> (w669:dbl[])
                  n509 = control-ref of="Stop here"() -> (w667:refnum<vi>)
                  n510 = call "MoveSinglePIMotor_Mercury.vi"("System no."=w678, "Axes to move"=w662, 3:"Move"=w669, "error in"=w665, 11:"Move"=TRUE ("Move"), "Stop refnum"=w667) -> ("error out"=w675:errorcluster)  [unwired: 12 in, 1 out]
                  n511 = Unbundle By Name(w675) -> ("status"=w676:bool)
                  n512 = case shown="False" w676 {
                    tunnel: w678 -> [w686 w697]
                    tunnel: [w684 w695] -> w677
                    tunnel: w675 -> [w688 _]
                    tunnel: w662 -> [w687 _]
                    frame False {
                      n513 = call "POS?.vi"("System no."=w686, "Axes to query"=w687, "error in"=w688) -> ("Position"=w685:dbl[], "error out"=w684:errorcluster)  [unwired: 15 in]
                      n514 = local write "Ligne à retard prête?"(TRUE ("Ligne à retard prête?")) -> ()
                      n515 = Index Array(array=w685) -> (element=w691:dbl)  [unwired: 1 in]
                      n516 = property on="Stop here" class="Bool (strict)"("Value"=FALSE ("Stop here")) -> ()  [unwired: 2 in, 2 out]
                      n517 = local write "Position ligne à retard"(w685) -> ()
                      n518 = local write "Position de la ligne à retard"(w691) -> ()
                    }
                    frame True {
                      n519 = call "ERR?.vi"("System no."=w697) -> ("error out"=w696:errorcluster)  [unwired: 17 in, 1 out]
                      n520 = property on="Stop here" class="Bool (strict)"("Value"=FALSE ("Stop here")) -> ()  [unwired: 2 in, 2 out]
                      n521 = local write "Ligne à retard prête?"(TRUE ("Ligne à retard prête?")) -> ()
                      n522 = call "GCSTranslateError.vi"("error in"=w696) -> ("Error Description"=w694:string, "error out"=w695:errorcluster)  [unwired: 16 in, 1 out]
                      n523 = local write "Error Description (delay line)"(w694) -> ()
                    }
                  }
                  n524 = local write "error out \nligne à retard"(w677) -> ()
                }
                event "zero à :": Value Change {
                  n525 = event-data() -> ()  [unwired: 1 in, 6 out]
                  n526 = Two Button Dialog(message="Voulez-vous vraiment changer le zéro?", 1:"Non" ("F button name (\"Cancel\")"), 2:"Oui" ("T button name (\"OK\")")) -> (T button?=w699:bool)
                  n527 = case shown="True" w699 {
                    frame False {
                    }
                    frame True {
                      n528 = local read "Fichier zéro ligne à retard"() -> (w710:path)
                      n529 = local read "zero"() -> (w704:dbl)
                      n530 = Open/Create/Replace File(file path (use dialog)=w710, operation (0:open)=T9."replace") -> (refnum out=w708:refnum<file>, error out=w707:errorcluster)  [unwired: 4 in, 1 out]
                      n531 = Format Into String(initial string=w708, error in=w707, w704) -> (resulting string=w705:refnum<file>, error out=w706:errorcluster)  [unwired: 1 in]
                      n532 = global write "Zero.vi" "Zero"(w704) -> ()
                      n533 = local write "Current zero position"(w704) -> ()
                      n534 = Close File(refnum=w705, error in=w706) -> (error out=w703:errorcluster)  [unwired: 1 out]
                      n535 = local write "error out\nLabview functions"(w703) -> ()
                    }
                  }
                }
                event "JOG - position": Value Change {
                  w715 = 2 ("System no.")
                  n536 = event-data() -> ()  [unwired: 1 in, 6 out]
                  n537 = local read "Step Size (mm)"() -> (w722:dbl)
                  n538 = local read "Position de la ligne à retard"() -> (w723:dbl)
                  n539 = local read "error out \nligne à retard"() -> (w719:errorcluster)
                  n540 = Subtract(x=w723, y=w722) -> (x-y=w721:dbl)
                  n541 = local read "Conn. \nAxes"() -> (w712:string[])
                  n542 = Build Array(w721) -> (w720:dbl[])
                  n543 = control-ref of="Stop here"() -> (w713:refnum<vi>)
                  n544 = call "MoveSinglePIMotor_Mercury.vi"("System no."=w715, "Axes to move"=w712, 3:"Move"=w720, "error in"=w719, 11:"Move"=TRUE ("Move"), "Stop refnum"=w713) -> ("Position"=w714:dbl[], "error out"=w716:errorcluster)  [unwired: 12 in]
                  n545 = Unbundle By Name(w716) -> ("status"=w717:bool)
                  n546 = case shown="False" w717 {
                    tunnel: w716 -> [w726 w736]
                    tunnel: w715 -> [w728 w735]
                    tunnel: w714 -> [_ _]
                    tunnel: w712 -> [w727 _]
                    frame False {
                      n547 = call "POS?.vi"("System no."=w728, "Axes to query"=w727, "error in"=w726) -> ("Position"=w724:dbl[], "error out"=w725:errorcluster)  [unwired: 15 in]
                      n548 = local write "error out \nligne à retard"(w725) -> ()
                      n549 = Index Array(array=w724) -> (element=w730:dbl)  [unwired: 1 in]
                      n550 = local write "Position ligne à retard"(w724) -> ()
                      n551 = local write "Position de la ligne à retard"(w730) -> ()
                      n552 = property on="Stop here" class="Bool (strict)"("Value"=FALSE ("Stop here")) -> ()  [unwired: 2 in, 2 out]
                    }
                    frame True {
                      n553 = call "ERR?.vi"("System no."=w735, "error in"=w736) -> ("error out"=w734:errorcluster)  [unwired: 16 in, 1 out]
                      n554 = call "GCSTranslateError.vi"("error in"=w734) -> ("Error Description"=w733:string, "error out"=w732:errorcluster)  [unwired: 16 in, 1 out]
                      n555 = local write "Error Description (delay line)"(w733) -> ()
                      n556 = local write "error out \nligne à retard"(w732) -> ()
                      n557 = property on="Stop here" class="Bool (strict)"("Value"=FALSE ("Stop here")) -> ()  [unwired: 2 in, 2 out]
                    }
                  }
                }
                event "JOG -delay": Value Change {
                  w744 = 2 ("System no.")
                  # "Division par deux à cause \nde l'aller-retour dans la ligne\nà retard"
                  n558 = event-data() -> ()  [unwired: 1 in, 6 out]
                  n559 = local read "Step Size (ps)"() -> (w755:dbl)
                  n560 = local read "error out \nligne à retard"() -> (w740:errorcluster)
                  n561 = local read "Position de la ligne à retard"() -> (w751:dbl)
                  n562 = Divide(x=w755, y=2.0) -> (x/y=w742:dbl)
                  n563 = Build Array(w742) -> (w754:dbl[])
                  n564 = call "SpaceTimeConversion.vi"("Conversion Type: T : Distance to Time\n                             F : Time to Distance"=FALSE ("Conversion Type: T : Distance to Time\n                             F : Time to Distance"), "Time IN (ps)"=w754, "Zero Position"=0.0) -> ("Time OUT (ps) / Distance OUT (mm)"=w752:dbl[])  [unwired: 1 in]
                  n565 = flat-sequence {
                    tunnel: w740 -> [w758]
                    tunnel: [w758] -> w739
                    frame #0 {
                      n566 = local write "Ligne à retard prête?"(FALSE ("Ligne à retard prête?")) -> ()
                    }
                  }
                  n567 = Index Array(array=w752) -> (element=w750:dbl)  [unwired: 1 in]
                  n568 = local read "Conn. \nAxes"() -> (w738:string[])
                  n569 = Subtract(x=w751, y=w750) -> (x-y=w749:dbl)
                  n570 = Build Array(w749) -> (w748:dbl[])
                  n571 = control-ref of="Stop here"() -> (w743:refnum<vi>)
                  n572 = call "MoveSinglePIMotor_Mercury.vi"("System no."=w744, "Axes to move"=w738, 3:"Move"=w748, "error in"=w739, 11:"Move"=TRUE ("Move"), "Stop refnum"=w743) -> ("error out"=w745:errorcluster)  [unwired: 12 in, 1 out]
                  n573 = Unbundle By Name(w745) -> ("status"=w746:bool)
                  n574 = case shown="False" w746 {
                    tunnel: w745 -> [w761 w773]
                    tunnel: w744 -> [w762 w772]
                    tunnel: w738 -> [w763 _]
                    frame False {
                      n575 = call "POS?.vi"("System no."=w762, "Axes to query"=w763, "error in"=w761) -> ("Position"=w759:dbl[], "error out"=w760:errorcluster)  [unwired: 15 in]
                      n576 = local write "error out \nligne à retard"(w760) -> ()
                      n577 = local write "Ligne à retard prête?"(TRUE ("Ligne à retard prête?")) -> ()
                      n578 = Index Array(array=w759) -> (element=w766:dbl)  [unwired: 1 in]
                      n579 = local write "Position ligne à retard"(w759) -> ()
                      n580 = local write "Position de la ligne à retard"(w766) -> ()
                      n581 = property on="Stop here" class="Bool (strict)"("Value"=FALSE ("Stop here")) -> ()  [unwired: 2 in, 2 out]
                    }
                    frame True {
                      n582 = call "ERR?.vi"("System no."=w772, "error in"=w773) -> ("error out"=w771:errorcluster)  [unwired: 16 in, 1 out]
                      n583 = local write "Ligne à retard prête?"(FALSE ("Ligne à retard prête?")) -> ()
                      n584 = call "GCSTranslateError.vi"("error in"=w771) -> ("Error Description"=w770:string, "error out"=w769:errorcluster)  [unwired: 16 in, 1 out]
                      n585 = local write "Error Description (delay line)"(w770) -> ()
                      n586 = local write "error out \nligne à retard"(w769) -> ()
                      n587 = property on="Stop here" class="Bool (strict)"("Value"=FALSE ("Stop here")) -> ()  [unwired: 2 in, 2 out]
                    }
                  }
                }
                event "Go delay": Value Change {
                  n588 = event-data() -> ()  [unwired: 1 in, 6 out]
                  n589 = stacked-sequence {
                    frame #0 {
                      n590 = local write "Ligne à retard prête?"(FALSE ("Ligne à retard prête?")) -> ()
                    }
                    frame #1 {
                      w782 = 2 ("System no.")
                      # "Division par 2 à cause de \nl'aller-retour dans la ligne \nà retard"
                      n591 = local read "Delay to reach"() -> (w779:dbl)
                      n592 = Divide(x=w779, y=2.0) -> (x/y=w777:dbl)
                      n593 = local read "error out \nligne à retard"() -> (w786:errorcluster)
                      n594 = global read "Zero.vi" "Zero"() -> (w790:dbl)
                      n595 = Build Array(w777) -> (w788:dbl[])
                      n596 = local read "Conn. \nAxes"() -> (w776:string[])
                      n597 = call "SpaceTimeConversion.vi"("Conversion Type: T : Distance to Time\n                             F : Time to Distance"=FALSE ("Conversion Type: T : Distance to Time\n                             F : Time to Distance"), "Time IN (ps)"=w788, "Zero Position"=w790) -> ("Time OUT (ps) / Distance OUT (mm)"=w787:dbl[])  [unwired: 1 in]
                      n598 = control-ref of="Stop here"() -> (w781:refnum<vi>)
                      n599 = call "MoveSinglePIMotor_Mercury.vi"("System no."=w782, "Axes to move"=w776, 3:"Move"=w787, "error in"=w786, 11:"Move"=TRUE ("Move"), "Stop refnum"=w781) -> ("Position"=w785:dbl[], "error out"=w783:errorcluster)  [unwired: 12 in]
                      n600 = Unbundle By Name(w783) -> ("status"=w784:bool)
                      n601 = case shown="False" w784 {
                        tunnel: w785 -> [_ _]
                        tunnel: w783 -> [w793 w805]
                        tunnel: w782 -> [w795 w804]
                        tunnel: w776 -> [w794 _]
                        frame False {
                          n602 = call "POS?.vi"("System no."=w795, "Axes to query"=w794, "error in"=w793) -> ("Position"=w791:dbl[], "error out"=w792:errorcluster)  [unwired: 15 in]
                          n603 = local write "Ligne à retard prête?"(TRUE ("Ligne à retard prête?")) -> ()
                          n604 = property on="Stop here" class="Bool (strict)"("Value"=FALSE ("Stop here")) -> ()  [unwired: 2 in, 2 out]
                          n605 = local write "error out \nligne à retard"(w792) -> ()
                          n606 = Index Array(array=w791) -> (element=w798:dbl)  [unwired: 1 in]
                          n607 = local write "Position ligne à retard"(w791) -> ()
                          n608 = local write "Position de la ligne à retard"(w798) -> ()
                        }
                        frame True {
                          n609 = call "ERR?.vi"("System no."=w804, "error in"=w805) -> ("error out"=w803:errorcluster)  [unwired: 16 in, 1 out]
                          n610 = property on="Stop here" class="Bool (strict)"("Value"=FALSE ("Stop here")) -> ()  [unwired: 2 in, 2 out]
                          n611 = call "GCSTranslateError.vi"("error in"=w803) -> ("Error Description"=w802:string, "error out"=w801:errorcluster)  [unwired: 16 in, 1 out]
                          n612 = local write "Ligne à retard prête?"(FALSE ("Ligne à retard prête?")) -> ()
                          n613 = local write "error out \nligne à retard"(w801) -> ()
                          n614 = local write "Error Description (delay line)"(w802) -> ()
                        }
                      }
                    }
                  }
                }
                event "Go pos": Value Change {
                  n615 = event-data() -> ()  [unwired: 1 in, 6 out]
                  n616 = stacked-sequence {
                    frame #0 {
                      n617 = local write "Ligne à retard prête?"(FALSE ("Ligne à retard prête?")) -> ()
                    }
                    frame #1 {
                      w809 = 2 ("System no.")
                      n618 = local read "Position à atteindre"() -> (w816:dbl)
                      n619 = local read "error out \nligne à retard"() -> (w814:errorcluster)
                      n620 = local read "Conn. \nAxes"() -> (w808:string[])
                      n621 = Build Array(w816) -> (w815:dbl[])
                      n622 = control-ref of="Stop here"() -> (w810:refnum<vi>)
                      n623 = call "MoveSinglePIMotor_Mercury.vi"("System no."=w809, "Axes to move"=w808, 3:"Move"=w815, "error in"=w814, 11:"Move"=TRUE ("Move"), "Stop refnum"=w810) -> ("error out"=w811:errorcluster)  [unwired: 12 in, 1 out]
                      n624 = Unbundle By Name(w811) -> ("status"=w812:bool)
                      n625 = case shown="False" w812 {
                        tunnel: w811 -> [w821 w831]
                        tunnel: w809 -> [w819 _]
                        tunnel: w808 -> [w820 _]
                        frame False {
                          n626 = call "POS?.vi"("System no."=w819, "Axes to query"=w820, "error in"=w821) -> ("Position"=w818:dbl[], "error out"=w817:errorcluster)  [unwired: 15 in]
                          n627 = local write "error out \nligne à retard"(w817) -> ()
                          n628 = local write "Ligne à retard prête?"(TRUE ("Ligne à retard prête?")) -> ()
                          n629 = Index Array(array=w818) -> (element=w824:dbl)  [unwired: 1 in]
                          n630 = property on="Stop here" class="Bool (strict)"("Value"=FALSE ("Stop here")) -> ()  [unwired: 2 in, 2 out]
                          n631 = local write "Position de la ligne à retard"(w824) -> ()
                          n632 = local write "Position ligne à retard"(w818) -> ()
                        }
                        frame True {
                          n633 = property on="Stop here" class="Bool (strict)"("Value"=FALSE ("Stop here")) -> ()  [unwired: 2 in, 2 out]
                          n634 = call "ERR?.vi"("System no."=2, "error in"=w831) -> ("error out"=w830:errorcluster)  [unwired: 16 in, 1 out]
                          n635 = call "GCSTranslateError.vi"("error in"=w830) -> ("Error Description"=w828:string, "error out"=w829:errorcluster)  [unwired: 16 in, 1 out]
                          n636 = local write "Ligne à retard prête?"(FALSE ("Ligne à retard prête?")) -> ()
                          n637 = local write "error out \nligne à retard"(w829) -> ()
                          n638 = local write "Error Description (delay line)"(w828) -> ()
                        }
                      }
                    }
                  }
                }
                event "Query Velocity": Value Change {
                  w833 = 2 ("System no.")
                  n639 = event-data() -> ()  [unwired: 1 in, 6 out]
                  n640 = local read "error out \nligne à retard"() -> (w837:errorcluster)
                  n641 = local read "Conn. \nAxes"() -> (w838:string[])
                  n642 = call "VEL?.vi"("System no."=w833, "Axes to query"=w838, "error in"=w837) -> ("Velocity"=w836:dbl[], "error out"=w834:errorcluster)  [unwired: 15 in]
                  n643 = Unbundle By Name(w834) -> ("status"=w835:bool)
                  n644 = case shown="False" w835 {
                    tunnel: w836 -> [w840 _]
                    tunnel: w834 -> [_ w844]
                    tunnel: w833 -> [_ w845]
                    frame False {
                      n645 = Index Array(array=w840) -> (element=w839:dbl)  [unwired: 1 in]
                      n646 = local write "Current velocity"(w839) -> ()
                    }
                    frame True {
                      n647 = call "ERR?.vi"("System no."=w845, "error in"=w844) -> ("error out"=w843:errorcluster)  [unwired: 16 in, 1 out]
                      n648 = call "GCSTranslateError.vi"("error in"=w843) -> ("Error Description"=w842:string, "error out"=w841:errorcluster)  [unwired: 16 in, 1 out]
                      n649 = local write "error out \nligne à retard"(w841) -> ()
                      n650 = local write "Error Description (delay line)"(w842) -> ()
                    }
                  }
                }
                event "zero ici": Value Change {
                  n651 = event-data() -> ()  [unwired: 1 in, 6 out]
                  n652 = stacked-sequence {
                    seq-local: [w847 _] -> [_ w852]
                    frame #0 {
                      n653 = local read "error out \nligne à retard"() -> (w849:errorcluster)
                      n654 = local read "Conn. \nAxes"() -> (w850:string[])
                      n655 = call "POS?.vi"("System no."=2, "Axes to query"=w850, "error in"=w849) -> ("Position"=w847:dbl[], "error out"=w848:errorcluster)  [unwired: 15 in]
                      n656 = local write "Position ligne à retard"(w847) -> ()
                      n657 = local write "error out \nligne à retard"(w848) -> ()
                    }
                    frame #1 {
                      n658 = Two Button Dialog(message="Voulez-vous remplacer le zéro?", 1:"Non" ("F button name (\"Cancel\")"), 2:"Oui" ("T button name (\"OK\")")) -> (T button?=w853:bool)
                      n659 = case shown="True" w853 {
                        tunnel: w852 -> [_ w865]
                        frame False {
                        }
                        frame True {
                          n660 = Index Array(array=w865) -> (element=w859:dbl)  [unwired: 1 in]
                          n661 = local read "Fichier zéro ligne à retard"() -> (w864:path)
                          n662 = global write "Zero.vi" "Zero"(w859) -> ()
                          n663 = local write "Current zero position"(w859) -> ()
                          n664 = Open/Create/Replace File(file path (use dialog)=w864, error in=errorcluster {"status"=FALSE, "code"=0, "source"=""}, operation (0:open)=T9."replace") -> (refnum out=w863:refnum<file>, error out=w861:errorcluster)  [unwired: 3 in, 1 out]
                          n665 = Format Into String(initial string=w863, error in=w861, w859) -> (resulting string=w858:refnum<file>, error out=w857:errorcluster)  [unwired: 1 in]
                          n666 = Close File(refnum=w858, error in=w857) -> ()  [unwired: 2 out]
                        }
                      }
                    }
                  }
                }
                event "Set Velocity": Value Change {
                  n667 = event-data() -> ()  [unwired: 1 in, 6 out]
                  n668 = local read "Set Vel."() -> (w867:dbl)
                  n669 = local read "Conn. \nAxes"() -> (w874:string[])
                  n670 = local read "error out \nligne à retard"() -> (w871:errorcluster)
                  n671 = Build Array(w867) -> (w873:dbl[])
                  n672 = call "VEL.vi"("System no."=2, "Axes to set"=w874, "Velocity values"=w873, "No.of digits"=i16 4, "error in"=w871) -> ("error out"=w870:errorcluster)  [unwired: 13 in, 1 out]
                  n673 = Unbundle By Name(w870) -> ("status"=w869:bool)
                  n674 = case shown="False" w869 {
                    tunnel: w870 -> [w877 w881]
                    tunnel: [w877 w879] -> w868
                    tunnel: w867 -> [w876 _]
                    frame False {
                      n675 = local write "Current velocity"(w876) -> ()
                    }
                    frame True {
                      n676 = call "ERR?.vi"("System no."=2, "error in"=w881) -> ("error out"=w880:errorcluster)  [unwired: 16 in, 1 out]
                      n677 = call "GCSTranslateError.vi"("error in"=w880) -> ("Error Description"=w878:string, "error out"=w879:errorcluster)  [unwired: 16 in, 1 out]
                      n678 = local write "Error Description (delay line)"(w878) -> ()
                    }
                  }
                  n679 = local write "error out \nligne à retard"(w868) -> ()
                }
                event "stop": Value Change {
                  w883 = TRUE
                  n680 = event-data() -> ()  [unwired: 1 in, 6 out]
                }
              }
            }
          }
        }
      }
    }
    n681 = Wait Until Next ms Multiple(millisecond multiple=u32 100 ("attente (ms)")) -> ()  [unwired: 1 out]
    n682 = Or(x="stop", y=w29) -> (x .or. y?=w31:bool)
    "INIT" <- w27
  }
  n683 = while {
    tunnel: [errorcluster {"status"=FALSE, "code"=0, "source"=""} ("error in (no error)")] -> w8
    tunnel: w3 -> [w886]
    tunnel: w2 -> [w885]
    stop <- w890 stop-if-true
    n684 = property on="Envoi cmde PilMot?" class="Bool (strict)"() -> ("Value"=w888:bool)  [unwired: 2 in, 2 out]
    n685 = Wait Until Next ms Multiple(millisecond multiple=u32 100) -> ()  [unwired: 1 out]
    n686 = case shown="False" w888 {
      tunnel: w886 -> [w909 _]
      tunnel: w885 -> [w908 _]
      frame False {
        # "Mise à jour de la position\ndes moteurs uniquement \nsi aucune commande n'est \nen cours d'envoi"
        n687 = shared-variable "My Computer\\OPC.lvlib\\Axe1_PositionTheorique"() -> (w914:i32)  [unwired: 1 in, 1 out]
        n688 = shared-variable "My Computer\\OPC.lvlib\\Axe2_PositionTheorique"() -> (w915:i32)  [unwired: 1 in, 1 out]
        n689 = shared-variable "My Computer\\OPC.lvlib\\Axe3_PositionTheorique"() -> (w916:i32)  [unwired: 1 in, 1 out]
        n690 = shared-variable "My Computer\\OPC.lvlib\\Axe4_PositionTheorique"() -> (w917:i32)  [unwired: 1 in, 1 out]
        n691 = shared-variable "My Computer\\OPC.lvlib\\Axe5_PositionTheorique"() -> (w918:i32)  [unwired: 1 in, 1 out]
        n692 = shared-variable "My Computer\\OPC.lvlib\\Axe6_PositionTheorique"() -> (w919:i32)  [unwired: 1 in, 1 out]
        n693 = local read "Positons Moteurs"() -> (w910:dbl[])
        n694 = local read "Coeff µm/pas"() -> (w912:dbl[])
        n695 = Insert Into Array(array=w910, index=0, new element #1=w914, new element #2=w915, new element #3=w916, new element #4=w917, new element #5=w918, new element #6=w919) -> (w907:dbl[])
        n696 = for {
          tunnel: w909 -> [w923] mode=indexing
          tunnel: w908 -> [w922] mode=indexing
          tunnel: w907 -> [w921] mode=indexing
          n697 = To Long Integer(number=w921) -> (32bit integer=w925:i32)
          n698 = To Long Integer(number=w921) -> (32bit integer=w924:i32)
          n699 = Less Or Equal?(x=w925, y=w923) -> (x <= y?=w928:bool)
          n700 = Greater Or Equal?(x=w924, y=w922) -> (x >= y?=w927:bool)
          n701 = Or(x=w928, y=w927) -> (x .or. y?=w926:bool)
          n702 = case shown="False" w926 {
            frame False {
            }
            frame True {
              n703 = call "Arret Urgence.vi"() -> ("error out"=w929:errorcluster)  [unwired: 11 in]
              n704 = local write "error out\nesbim"(w929) -> ()
            }
          }
        }
        n705 = call "ConvertStepsmm.vi"("Conversion: T: pas->mm\n                      F: mm->pas"=TRUE ("Conversion"), "Input en pas"=w907, "Facteur de conversion\n en µm/pas"=w912) -> ("Output en mm"=→"Positons Moteurs":dbl[])  [unwired: 7 in, 1 out]
      }
      frame True {
      }
    }
    n706 = property on="Referencing..." class="Bool (strict)"() -> ("Blinking"=w884:bool)  [unwired: 2 in, 2 out]
    n707 = case shown="False" w884 {
      frame False {
        n708 = stacked-sequence {
          frame #0 {
            n709 = local read "Initialisation OK?"() -> (w891:bool)
            n710 = case shown="False" w891 {
              frame False {
              }
              frame True {
                n711 = local read "Axes \nConn."() -> (w895:string[])
                n712 = call "#5.vi"("System no."=1) -> ("Axis moving?"=w898:bool[], "error out"=w896:errorcluster)  [unwired: 17 in]
                n713 = property on="Axe en MVT" class="Arr (strict)"("Value"=w898) -> ()  [unwired: 2 in, 2 out]
                n714 = call "POS?.vi"("System no."=1, "Axes to query"=w895, "error in"=w896) -> ("Position"=w894:dbl[], "error out"=w893:errorcluster)  [unwired: 15 in]
                n715 = local write "Position Moteurs (PI)"(w894) -> ()
                n716 = local write "error out \nPI Enceinte"(w893) -> ()
              }
            }
          }
          frame #1 {
            n717 = local read "Initialisation OK? 2"() -> (w899:bool)
            n718 = case shown="False" w899 {
              frame False {
              }
              frame True {
                n719 = local read "Axes \nConn. 2"() -> (w905:string[])
                n720 = call "#5.vi"("System no."=2) -> ("Axis moving?"=w901:bool[], "error out"=w902:errorcluster)  [unwired: 17 in]
                n721 = property on="Axe en MVT 2" class="Arr (strict)"("Value"=w901) -> ()  [unwired: 2 in, 2 out]
                n722 = call "POS?.vi"("System no."=2, "Axes to query"=w905, "error in"=w902) -> ("Position"=w900:dbl[], "error out"=w904:errorcluster)  [unwired: 15 in]
                n723 = local write "Position Moteurs (PI) 2"(w900) -> ()
                n724 = local write "error out \nPI Enceinte 2"(w904) -> ()
                n725 = local write "Position 2"(w900) -> ()
              }
            }
          }
        }
      }
      frame True {
      }
    }
    n726 = property on="stop" class="Bool (strict)"() -> ("Value"=w890:bool)  [unwired: 2 in, 2 out]
  }
  n727 = property on="stop" class="Bool (strict)"(error in=w8, "Value"=FALSE ("stop")) -> ()  [unwired: 1 in, 2 out]
